vi "RT.vi"() -> ()   [LabVIEW 2012]
uses:
  Type/_RT Instrument State.ctl
  Type/RT Loop Events.ctl
  Type/_RT Parameter.ctl
  Type/_RT Active Ch.ctl
  Type/_RT Expt.ctl
  Type/_Run Mode.ctl
  Type/_RT Mass Range.ctl
  Type/_RT Res Type.ctl
  Type/_LED States.ctl
  Type/_LCD Line1 Msg.ctl
  Type/_LCD Line2 Msg.ctl
  Type/_RT LED Num.ctl
  Type/_Pump Parameter.ctl
  Type/_RW Status.ctl
  Type/_RT Serial Command.ctl
  Type/_FPGA Indicator.ctl
  _RT Global.vi
  <vilib>/FPGAPlugInAG/sbRIO-9606/niLvFpga_Open_sbRIO-9606.vi
  <vilib>/Utility/error.llb/Error Cluster From Error Code.vi
  <vilib>/rvi/errors/niLvFpgaAdjustHostInterfaceError.vi
  <vilib>/Utility/config.llb/Read Key (Boolean).vi
  <vilib>/Utility/config.llb/Read Key (String).vi
  <vilib>/Utility/config.llb/Write Key (Boolean).vi
  <vilib>/Utility/config.llb/Write Key (String).vi
  <vilib>/rvi/interface/nirviOpenFPGA/nirviOpenFPGA.xnode
  FPGA Bitfiles/FPGA9606.lvbitx
  <vilib>/rvi/interface/nirviMethod/nirviMethod.xnode
  <vilib>/rvi/interface/nirviReadWriteControl/nirviReadWriteControl.xnode
  <vilib>/Utility/config.llb/NI_LVConfig.lvlib
  <vilib>/NI_Real-Time Target Support.lvlib
  <vilib>/rvi/errors/niLvFpgaMergeErrorWithErrorCode.vi
  NiFpgaLv.dll
  <vilib>/FPGAPlugInAG/sbRIO-9606/niLvFpga_ConfigureFifo_sbRIO-9606.vi
  <vilib>/FPGAPlugInAG/sbRIO-9606/niLvFpga_StartFifo_sbRIO-9606.vi
panel:
  out "Disconnection#":u8
  out "Message Type":string
  out "Rt Loop Events":T1
  out "code":i32
  out "InstrState":T2=enum."Mass Spectrometer is Off"
  out "Fault":bool
  out "Ready":bool
  out "Running":bool
  out "RunMode":i32
  in  "RT Version":u32=965150731
  out "FPGA Version":u32
  out "Time (s)":dbl
  out "Connected?":bool
  # "Run  Status"
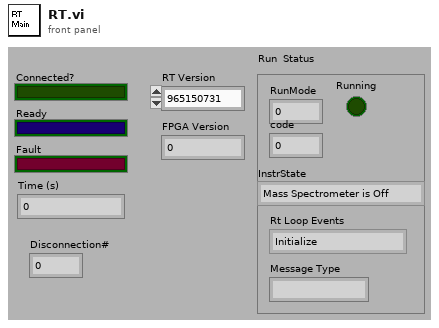
[diagram p1: front panel]
types:
  T1 = typedef "RT Loop Events.ctl" = enum16{"Initialize", "Wait for Connection", "Wait for Command", "Send Reply"}
  T2 = typedef "_RT Instrument State.ctl" = enum16{"Initializing", "Mass Spectrometer is Off", "Starting Up", "Turning Power Off", "Going to Standby", "Roughing Pump Ready", "Turning Turbo Off", "Turbo Startup", "Turbopump Ready", "Checking Vacuum", "Going to Ready", "Ready", "Running", "Source Standby", "Lost Communication", "Shutting Down", "Fault", "24V Standby", "Go to 24V Standby", "Turbopump Ready-Waiting"}
  T3 = typedef "_RT Parameter.ctl" = cluster{"RunMode":i32, "Initial Ch":T4[], "Sync":u8, "Expt":T5[], "EqTime(mS)":i32}
  T4 = typedef "_RT Active Ch.ctl" = cluster{"Start":i32, "Step":i32, "ChID":i32}
  T5 = typedef "_RT Expt.ctl" = cluster{"StartT(mS)":i32, "#Cycles":i32, "Scan Type":T6, "PauseT(uS)":i32, "Polarity":u8, "DelayT(mS)":i32, "Active Ch":T4[], "Mass Range":T7[]}
  T6 = typedef "_Run Mode.ctl" = enum16{"MRM (Q1/Q2)", "Q1 Scan", "Q1 SRM", "Q2 Scan", "Q2 SRM", "Product Scan", "Precursor Scan", "Neutral Loss", "Neutral Gain"}
  T7 = typedef "_RT Mass Range.ctl" = cluster{"Steps":i32, "Dwell(uS)":i32, "Resolution Type":T8, "Ramping Ch":T4[]}
  T8 = typedef "_RT Res Type.ctl" = u16
  T9 = typedef "Semaphore RefNum" = refnum<k1>
  T10 = typedef "_RT Instrument 2.ctl" = cluster{"Table":T11[], "Instrument":string[]}
  T11 = typedef "_RT Configuration 2.ctl" = cluster{"Name":string, "Ch#":u8, "Min":dbl, "Max":dbl, "Def+":dbl, "Def-":dbl, "Offset":dbl, "Slope":dbl, "Type":u8, "Description":string, "SettleT":dbl}
  T12 = cluster{"Rt Loop Events":T1, "Connection ID":refnum<k5>, "Parameter":T3, "Info":string, "Data Array":i32[], "error":errorcluster}
  T13 = typedef "_Pump Parameter.ctl" = enum16{"Turn Pump Motor On", "Turn Pump Motor Off", "Read Pump Oil Deficiency", "Read Rotation Switch Point Attained", "Read Ele. Drive Over Temperature", "Read Pump Over Temperature", "Read Set Rotation Speed Attained", "Read Turbopump Accelerates", "Read Actual Rotation Speed in Hz", "Read Motor Current in A", "Read Operating Hours in h", "Read Motor Voltage in V", "Read Motor Power in W", "Set Rotation Speed Switchpoint in %", "Clear Error", "Read Error Code", "Read Bearing Temperature", "Read Hardware Version", "Read Firmware Version", "Read Operating Hours (Drive)", "Read Rotational Speed (rpm)", "Read Power Stage Temperature", "Read Electronics Temperature", "Read Upper Pump Temperature", "Read Motor Temperature", "Read Error Code History, 1", "Read Error Code History, 2", "Read Error Code History, 3", "Read Error Code History, 4", "Read Error Code History, 5", "Read Error Code History, 6", "Read Error Code History, 7", "Read Error Code History, 8", "Read Error Code History, 9", "Read Error Code History, 10"}
  T14 = typedef "_RW Status.ctl" = enum8{"Done", "Do Read", "Do Write", "Set Latch1", "Set Latch2", "Set Latch3", "Set Latch4", "RP ON", "EL ON", "Serial Send", "Set LC Out", "Get LC In", "Read VAC", "Table Test", "Get Interlock", "Do Read2", "Do Write2"}
  T15 = typedef "_RT Serial Command.ctl" = cluster{"Port Type":u16, "baud rate (9600)":u32, "data bits (8)":u16, "stop bits (1)":u16, "parity (0:none)":u16, "DoRead":bool, "Command":string}
  T16 = typedef "_FPGA Indicator.ctl" = enum16{"Done", "Ready", "Count Available", "SendSerial", "LED State"}
  T17 = typedef "NI_LVConfig.lvlib/Config Data RefNum.ctl" = refnum<k1>
  T18 = typedef "_RT Startup Options.ctl" = cluster{"Door":bool, "Curtain":bool, "Pressure":bool, "Turbo":bool, "SysPoll":bool, "GasFlag":bool}
  T19 = cluster{"Info":string, "Data Array":i32[], "error":errorcluster}
  T20 = typedef "_RT LED Num.ctl" = enum8{"ReadKey", "ClearKeyBuffer", "ClearLCD", "BacklightOn"}
  T21 = typedef "_LED States.ctl" = enum8{"Idle", "Solid B", "Solid R", "Solid P", "Off B", "Off R", "Off P", "Off BRP", "Off RP", "Flash R&P", "Flash P"}
  T22 = typedef "_LCD Line2 Msg.ctl" = u16
  T23 = typedef "_LCD Line1 Msg.ctl" = u16
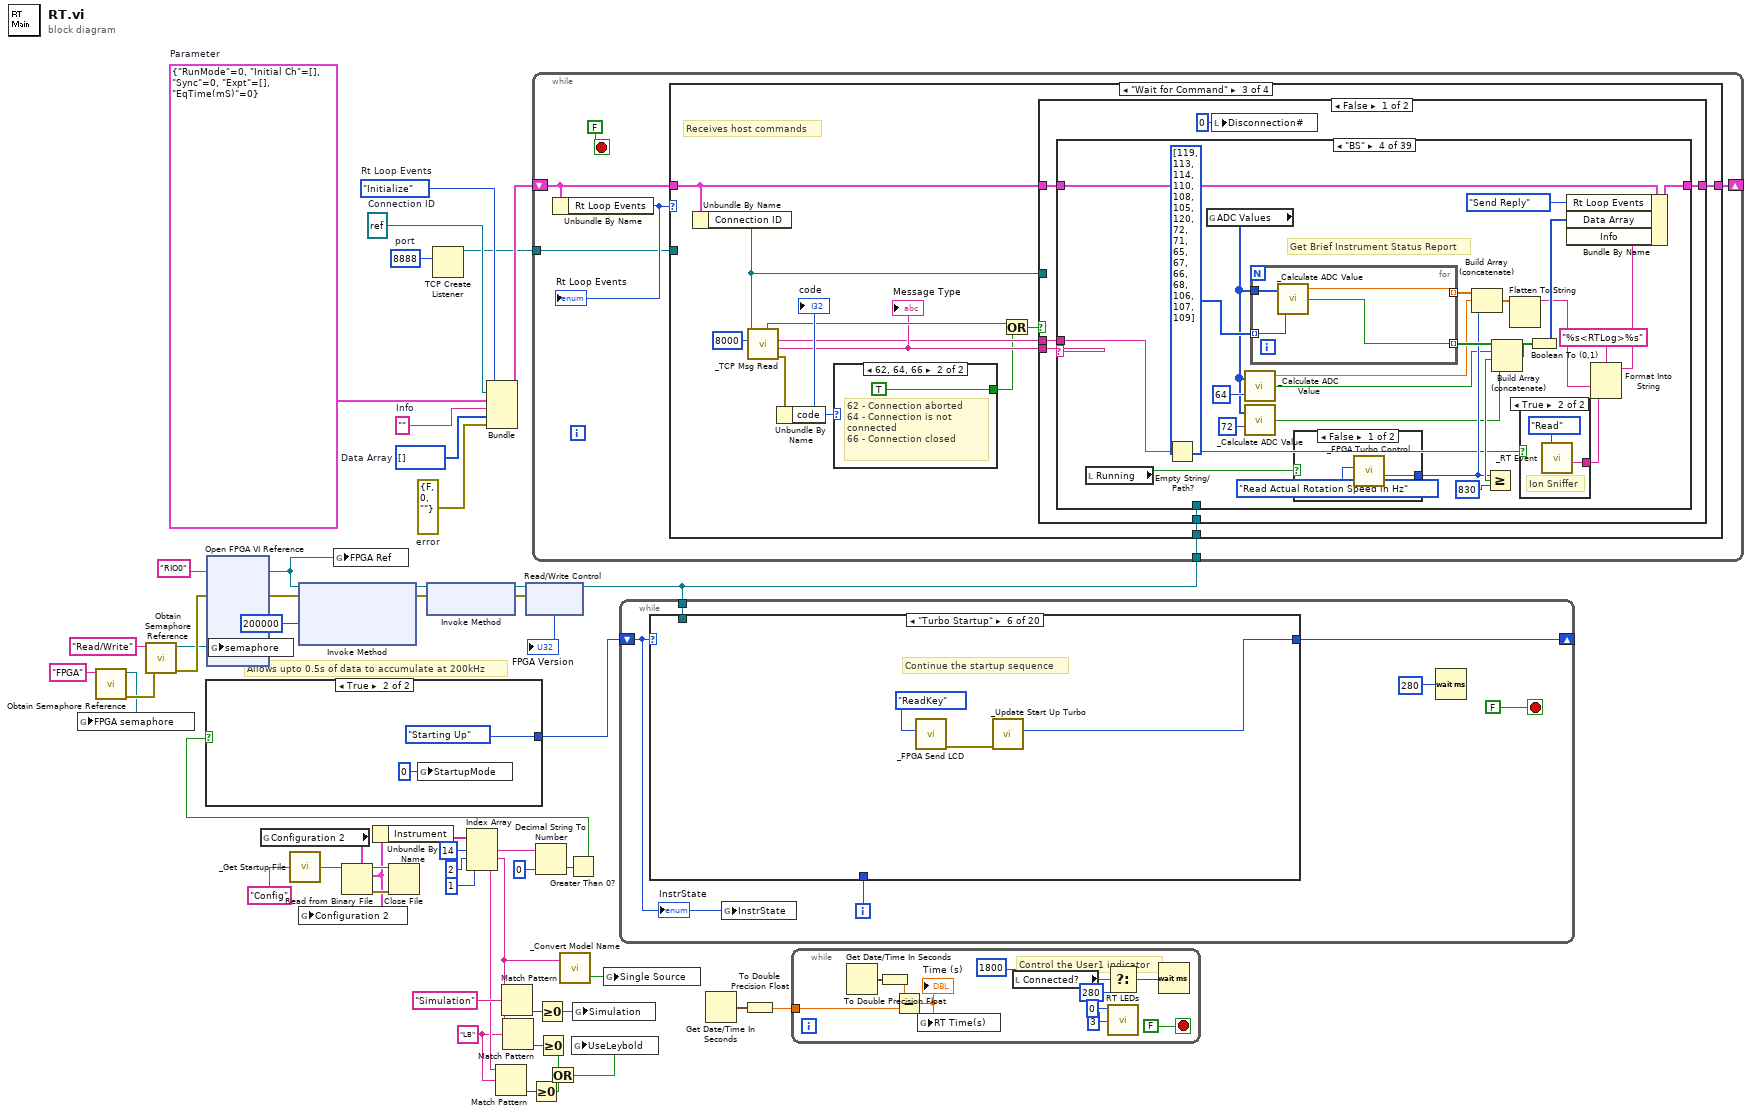
[diagram p0: block diagram]
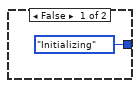
[diagram p2: hidden frame]
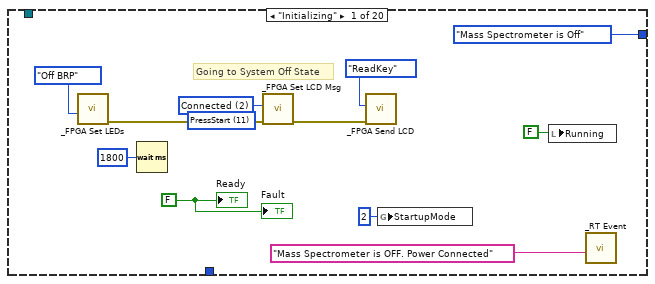
[diagram p3: hidden frame]
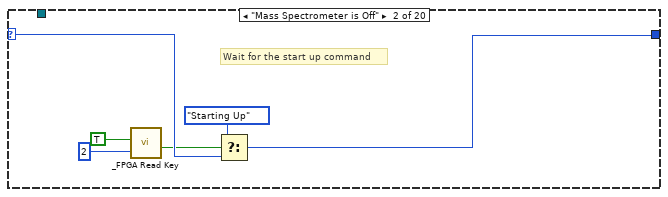
[diagram p4: hidden frame]
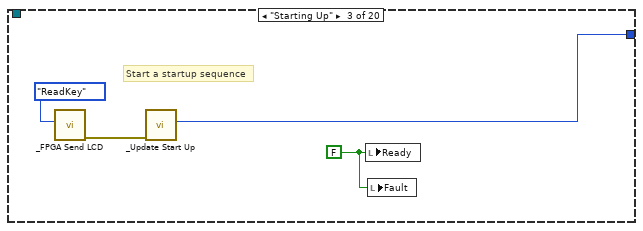
[diagram p5: hidden frame]
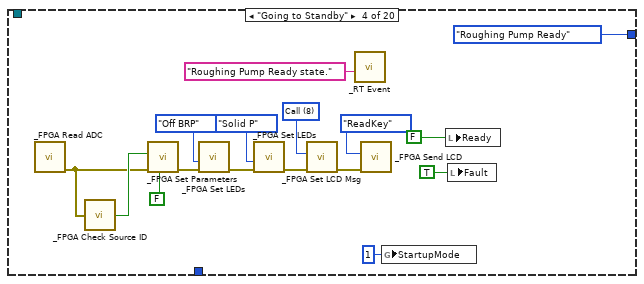
[diagram p6: hidden frame]
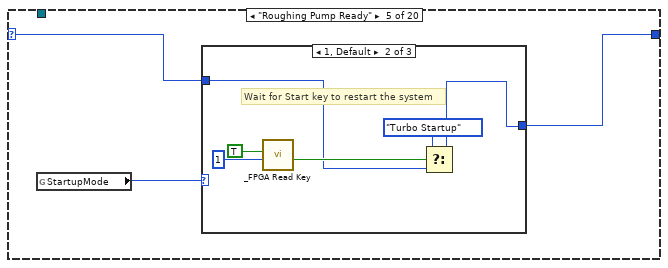
[diagram p7: hidden frame]
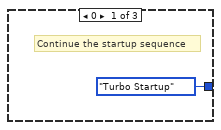
[diagram p8: hidden frame]
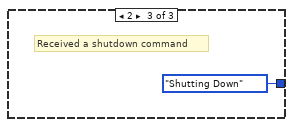
[diagram p9: hidden frame]
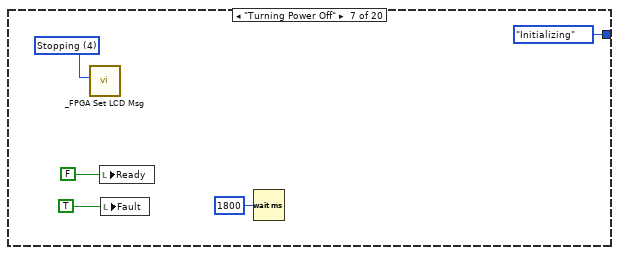
[diagram p10: hidden frame]
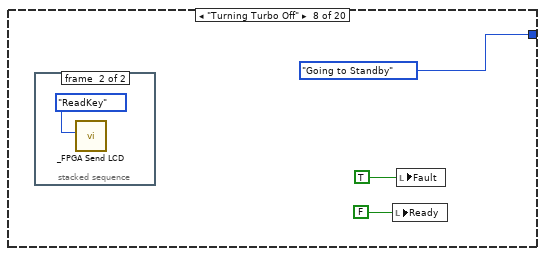
[diagram p11: hidden frame]
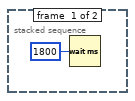
[diagram p12: hidden frame]
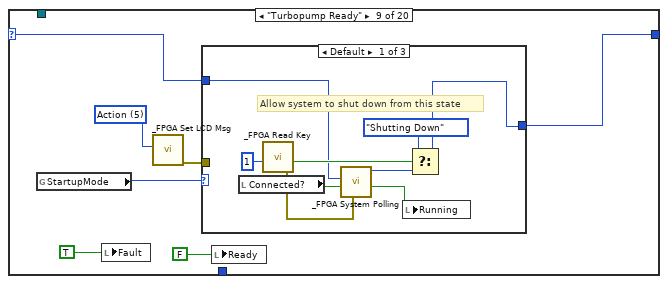
[diagram p13: hidden frame]
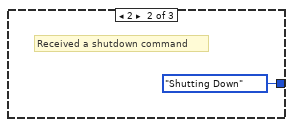
[diagram p14: hidden frame]
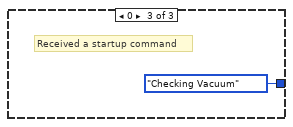
[diagram p15: hidden frame]
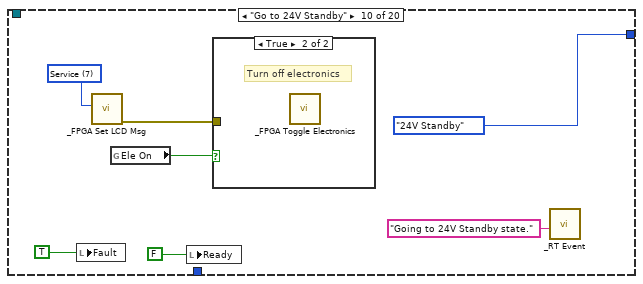
[diagram p16: hidden frame]
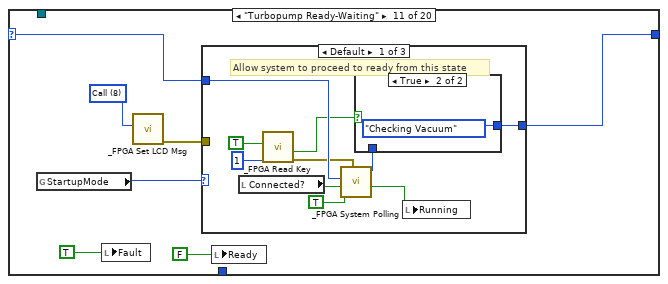
[diagram p18: hidden frame]
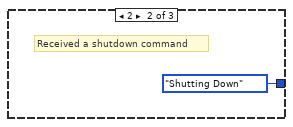
[diagram p20: hidden frame]
diagram:
  w4 = "LB" ("regular expression")
  w39 = T3 {"RunMode"=0, "Initial Ch"=[], "Sync"=0, "Expt"=[], "EqTime(mS)"=0}  # Parameter
  w41 = u16 8888  # port
  w49 = i32[] []  # Data Array
  w50 = ""  # Info
  w51 = errorcluster {"status"=FALSE, "code"=0, "source"=""}  # error
  w53 = refnum<k5> refnum  # Connection ID
  w54 = RT_Loop_Events."Initialize"  # Rt Loop Events
  # "Allows upto 0.5s of data to accumulate at 200kHz"
  n1 = call <vilib>:"Obtain Semaphore Reference.vi"("name (unnamed)"="FPGA") -> ("error out"=w23:errorcluster, "semaphore"=w21:T9)  [unwired: 2 in, 3 out]
  n2 = global write "_RT Global.vi" "FPGA semaphore"(w21) -> ()
  n3 = call <vilib>:"Obtain Semaphore Reference.vi"("error in (no error)"=w23, "name (unnamed)"="Read/Write") -> ("error out"=w26:errorcluster, "semaphore"=w25:T9)  [unwired: 1 in, 3 out]
  n4 = xnode "Open FPGA VI Reference"("error in"=w26, "resource name"="RIO0") -> ("FPGA VI Reference Out"=w12:refnum<k20>, "error out"=w43:errorcluster)
  n5 = global write "_RT Global.vi" "semaphore"(w25) -> ()
  n6 = global read "_RT Global.vi" "Configuration 2"() -> (w37:T10)
  n7 = call "_Get Startup File.vi"("FileName"="Config" ("key")) -> ("FilePath"=w11:path)
  n8 = xnode "Invoke Method"("FPGA VI Reference In"=w12, "error in"=w43, "Requested Depth"=u32 200000 ("Depth")) -> ("FPGA VI Reference Out"=w45:refnum<k20>, "error out"=w46:errorcluster)  [unwired: 1 out]
  n9 = global write "_RT Global.vi" "FPGA Ref"(w12) -> ()
  n10 = Read from Binary File(5:w37, 11:w11) -> (0:w36:errorcluster, 2:w34:T10, 3:w35:refnum<file>)  [unwired: 1 in, 4 out]
  n11 = global write "_RT Global.vi" "Configuration 2"(w34) -> ()
  n12 = Unbundle By Name(w34) -> ("Instrument"=w33:string[])
  n13 = Close File(refnum=w35, error in=w36) -> ()  [unwired: 2 out]
  n14 = xnode "Invoke Method"("FPGA VI Reference In"=w45, "error in"=w46) -> ("FPGA VI Reference Out"=w47:refnum<k20>, "error out"=w48:errorcluster)
  n15 = TCP Create Listener(10:w41) -> (3:w40:refnum<k5>)  [unwired: 1 in, 5 out]
  n16 = Index Array(array=w33, index #1=14 ("index"), index #2=2 ("index"), index #3=1 ("index")) -> (element #1=w30:string, element #2=w8:string, element #3=w5:string)
  n17 = Bundle("Rt Loop Events"=w54, "Connection ID"=w53, "Parameter"=w39, "Info"=w50, "Data Array"=w49, "error"=w51) -> (w52:T12)  [unwired: 1 out]
  n18 = Match Pattern(string=w5, regular expression=w4) -> (offset past match=w6:i32)  [unwired: 4 out]
  n19 = Match Pattern(string=w8, regular expression="Simulation") -> (offset past match=w19:i32)  [unwired: 4 out]
  n20 = Match Pattern(string=w8, regular expression=w4) -> (offset past match=w9:i32)  [unwired: 4 out]
  n21 = xnode "Read/Write Control"("FPGA VI Reference In"=w47, "error in"=w48) -> ("FPGA VI Reference Out"=w15:refnum<k20>, "Version"=→"FPGA Version":u32)  [unwired: 1 out]
  n22 = Greater Or Equal To 0?(x=w6) -> (x >= 0?=w2:bool)
  n23 = while {
    shift-right: [w57] -> _
    shift-left: w52 -> [w58]
    tunnel: w15 -> [w56]
    tunnel: w40 -> [w55]
    stop <- FALSE stop-if-true
    n24 = Unbundle By Name(w58) -> ("Rt Loop Events"=w59:T1)
    "Rt Loop Events" <- w59
    n25 = case shown="\"Wait for Command\"" w59 {
      tunnel: w58 -> [w85 w126 w146 w778]
      tunnel: [w84 w125 w145 w777] -> w57
      tunnel: w56 -> [_ _ w141 _]
      tunnel: w55 -> [_ w123 _ _]
      frame "Initialize", Default {
        w63 = FALSE ("Connected?")
        w78 = FALSE ("Connected?")
        w73 = "RT" ("section")
        # "Initialize All Instrument Parameters"
        n26 = stacked-sequence {
          frame #0 {
            n27 = call "_Read RT Table.vi"("key"="Cal") -> ("Table"=w87:dbl[][])  [unwired: 2 in, 4 out]
            n28 = global write "_RT Global.vi" "Q1 Cal"(w87) -> ()
            n29 = call "_Read RT Table.vi"("key"="Cal2") -> ("Table"=w88:dbl[][])  [unwired: 2 in, 4 out]
            n30 = global write "_RT Global.vi" "Q2 Cal"(w88) -> ()
            n31 = call "_Read RT Table.vi"("key"="Cal3") -> ("Table"=w89:dbl[][])  [unwired: 2 in, 4 out]
            n32 = global write "_RT Global.vi" "Q1 -Cal"(w89) -> ()
            n33 = call "_Read RT Table.vi"("key"="Cal4") -> ("Table"=w90:dbl[][])  [unwired: 2 in, 4 out]
            n34 = global write "_RT Global.vi" "Q2 -Cal"(w90) -> ()
            n35 = call "_Read RT Table.vi"("key"="Res") -> ("Table"=w91:dbl[][])  [unwired: 2 in, 4 out]
            n36 = global write "_RT Global.vi" "Q1 Res Hi"(w91) -> ()
            n37 = call "_Read RT Table.vi"("key"="Res2") -> ("Table"=w92:dbl[][])  [unwired: 2 in, 4 out]
            n38 = global write "_RT Global.vi" "Q2 Res Hi"(w92) -> ()
            n39 = call "_Read RT Table.vi"("key"="Res3") -> ("Table"=w93:dbl[][])  [unwired: 2 in, 4 out]
            n40 = global write "_RT Global.vi" "Q1 Res Med"(w93) -> ()
            n41 = call "_Read RT Table.vi"("key"="Res4") -> ("Table"=w94:dbl[][])  [unwired: 2 in, 4 out]
            n42 = global write "_RT Global.vi" "Q2 Res Med"(w94) -> ()
            n43 = call "_Read RT Table.vi"("key"="Res5") -> ("Table"=w95:dbl[][])  [unwired: 2 in, 4 out]
            n44 = global write "_RT Global.vi" "Q1 Res Lo"(w95) -> ()
            n45 = call "_Read RT Table.vi"("key"="Res6") -> ("Table"=w96:dbl[][])  [unwired: 2 in, 4 out]
            n46 = global write "_RT Global.vi" "Q2 Res Lo"(w96) -> ()
            n47 = call "_Read RT Table.vi"("key"="Res7") -> ("Table"=w97:dbl[][])  [unwired: 2 in, 4 out]
            n48 = global write "_RT Global.vi" "Q1 -Res Hi"(w97) -> ()
            n49 = call "_Read RT Table.vi"("key"="Res8") -> ("Table"=w98:dbl[][])  [unwired: 2 in, 4 out]
            n50 = global write "_RT Global.vi" "Q2 -Res Hi"(w98) -> ()
            n51 = call "_Read RT Table.vi"("key"="Res9") -> ("Table"=w99:dbl[][])  [unwired: 2 in, 4 out]
            n52 = global write "_RT Global.vi" "Q1 -Res Med"(w99) -> ()
            n53 = call "_Read RT Table.vi"("key"="Res10") -> ("Table"=w100:dbl[][])  [unwired: 2 in, 4 out]
            n54 = global write "_RT Global.vi" "Q2 -Res Med"(w100) -> ()
            n55 = call "_Read RT Table.vi"("key"="Res11") -> ("Table"=w101:dbl[][])  [unwired: 2 in, 4 out]
            n56 = global write "_RT Global.vi" "Q1 -Res Lo"(w101) -> ()
            n57 = call "_Read RT Table.vi"("key"="Res12") -> ("Table"=w102:dbl[][])  [unwired: 2 in, 4 out]
            n58 = global write "_RT Global.vi" "Q2 -Res Lo"(w102) -> ()
          }
          frame #1 {
            n59 = for {
              N: 16 -> [_]
              i -> [w120]
              n60 = call "_Update Cal or Res Data.vi"("Table Type"=w120) -> ()  [unwired: 2 in, 5 out]
            }
          }
        }
        n61 = call "_Get Startup File.vi"("FileName"="ADC" ("key")) -> ("FilePath"=w62:path)
        n62 = global read "_RT Global.vi" "ADC Table"() -> (w64:T11[])
        n63 = Read from Binary File(5:w64, 11:w62) -> (0:w66:errorcluster, 2:w65:T11[], 3:w67:refnum<file>)  [unwired: 1 in, 4 out]
        n64 = global write "_RT Global.vi" "ADC Table"(w65) -> ()
        n65 = Close File(refnum=w67, error in=w66) -> ()  [unwired: 2 out]
        n66 = Bundle By Name(cluster=w85, "Rt Loop Events"=RT_Loop_Events."Wait for Connection") -> (w84:T12)
        n67 = call "_RT Open Preference File.vi"() -> ("refnum"=w77:T17)  [unwired: 7 out]
        n68 = global read "_RT Global.vi" "StartupOptions"() -> (w68:T18)
        n69 = local write "Connected?"(w63) -> ()
        n70 = local write "Ready"(w63) -> ()
        n71 = call-poly <vilib>:"Read Key.vi"("section"=w73, "default value"=w78, "key"="Q1Pol", "refnum"=w77) -> ("value"=w79:bool, "refnum out"=w80:T17)  [unwired: 1 in, 5 out]
        n72 = local write "Fault"(w63) -> ()
        n73 = global write "_RT Global.vi" "IgnoreError"(w63) -> ()
        n74 = global write "_RT Global.vi" "Ele On"(w63) -> ()
        n75 = Flatten To String(anything=w68) -> (data string=w71:string)  [unwired: 1 in, 4 out]
        n76 = call-poly <vilib>:"Read Key.vi"("section"=w73, "default value"=w78, "key"="Q2Pol", "refnum"=w80) -> ("value"=w76:bool, "refnum out"=w75:T17)  [unwired: 1 in, 5 out]
        n77 = global write "_RT Global.vi" "Q2 POL"(w76) -> ()
        n78 = global write "_RT Global.vi" "Q1 POL"(w79) -> ()
        n79 = call-poly <vilib>:"Read Key.vi"("section"=w73, "default value"=w71, "key"="SUOpt", "refnum"=w75) -> ("value"=w70:string, "refnum out"=w72:T17)  [unwired: 2 in, 4 out]
        n80 = Unflatten From String(type=w68, binary string=w70) -> (value=w69:T18)  [unwired: 1 in, 4 out]
        n81 = global write "_RT Global.vi" "StartupOptions"(w69) -> ()
        n82 = call <vilib>:"Close Config Data.vi"("write file if changed (T)"=TRUE ("write configuration file? (T)"), "refnum"=w72) -> ()  [unwired: 1 in, 9 out]
      }
      frame "Wait for Connection" {
        # "Waits for new host connection"
        n83 = TCP Wait On Listener(9:-1 ("timeout ms (wait forever: -1)"), 11:w123) -> (0:w124:errorcluster, 4:w122:refnum<k5>)  [unwired: 1 in, 4 out]
        n84 = case shown="No Error" w124 {
          tunnel: w126 -> [w133 w136]
          tunnel: w122 -> [w130 _]
          tunnel: [w132 w134] -> w125
          frame No Error {
            n85 = local write "Disconnection#"(u8 0 ("Disconnection#")) -> ()
            n86 = local write "Connected?"(TRUE ("Connected?")) -> ()
            n87 = call "_RT Event.vi"("Event"="PC Communication Established") -> ()  [unwired: 2 in, 5 out]
            n88 = Bundle By Name(cluster=w133, "Connection ID"=w130, "Rt Loop Events"=RT_Loop_Events."Wait for Command") -> (w132:T12)
          }
          frame Error {
            n89 = Bundle By Name(cluster=w136, "Rt Loop Events"=RT_Loop_Events."Wait for Connection") -> (w134:T12)
          }
        }
      }
      frame "Wait for Command" {
        # "Receives host commands"
        n90 = Unbundle By Name(w146) -> ("Connection ID"=w138:refnum<k5>)
        n91 = call "_TCP Msg Read.vi"("timeout ms (10000)"=8000 ("millisecond multiple"), "connection ID"=w138) -> ("error out"=w140:errorcluster, "Message Type"=w144:string, "Data Stream"=w143:string, "Timed Out?"=w147:bool)  [unwired: 3 in, 3 out]
        "Message Type" <- w144
        n92 = Unbundle By Name(w140) -> ("code"=w148:i32)
        "code" <- w148
        n93 = case shown="62, 64, 66" w148 {
          tunnel: [_ TRUE ("abort (F)")] -> w137
          frame Default {
          }
          frame 62, 64, 66 {
            # "62 - Connection aborted\n64 - Connection is not connected\n66 - Connection closed"
          }
        }
        n94 = Or(x=w147, y=w137) -> (x .or. y?=w139:bool)
        n95 = case shown="False" w139 {
          tunnel: w146 -> [w153 w763]
          tunnel: [w152 w762] -> w145
          tunnel: w144 -> [w150 _]
          tunnel: w143 -> [w154 _]
          tunnel: w141 -> [w151 _]
          tunnel: w138 -> [_ w759]
          frame False {
            n96 = case shown="\"BS\"" w150 {
              selector: w150 -> [_ _ _ _ _ _ _ _ _ _ _ _ _ _ _ _ _ _ _ _ _ _ _ _ _ _ _ _ _ _ _ _ _ _ _ _ _ _ w755]
              tunnel: w154 -> [_ w171 w176 w189 w221 w230 w252 w272 _ w292 _ _ _ _ _ w360 _ w425 w449 w458 _ w464 w482 w490 w498 _ w507 w531 w546 _ w575 w578 w588 w608 w628 w644 w691 w705 _]
              tunnel: w153 -> [w159 w168 w181 w206 w224 w233 w249 w269 w286 w294 w300 w305 w314 w349 w357 w364 w422 w429 w452 w455 w462 w474 w479 w487 w495 w505 w512 w534 w544 w556 w572 w582 w595 w606 w626 w641 w701 w711 w751]
              tunnel: [w158 w167 w180 w205 w223 w232 w248 w268 w285 w293 w299 w304 w313 w348 w356 w363 w421 w428 w451 w454 w461 w473 w478 w486 w494 w504 w511 w533 w543 w555 w571 w581 w594 w605 w625 w640 w700 w708 w750] -> w152
              tunnel: w151 -> [_ _ _ _ _ _ _ _ _ _ _ _ w306 w345 _ _ w418 _ _ _ _ _ _ _ _ _ _ _ w542 _ _ _ w593 w604 w624 w637 w690 _ _]
              frame "AG" {
                # "Get ADC Table"
                n97 = global read "_RT Global.vi" "ADC Table"() -> (w156:T11[])
                n98 = Flatten To String(anything=w156) -> (data string=w155:string)  [unwired: 1 in, 4 out]
                n99 = Bundle By Name(cluster=w159, "Rt Loop Events"=RT_Loop_Events."Send Reply", "Info"=w155) -> (w158:T12)
              }
              frame "AS" {
                # "Set ADC Table"
                n100 = global read "_RT Global.vi" "ADC Table"() -> (w170:T11[])
                n101 = Unflatten From String(type=w170, binary string=w171) -> (value=w166:T11[], error out=w163:errorcluster)  [unwired: 1 in, 3 out]
                n102 = call "_Get Startup File.vi"("FileName"="ADC" ("key")) -> ("FilePath"=w161:path)
                n103 = global write "_RT Global.vi" "ADC Table"(w166) -> ()
                n104 = Write to Binary File(file (use dialog)=w161, data=w166, error in=w163) -> (refnum out=w164:refnum<file>, error out=w165:errorcluster)  [unwired: 4 out]
                n105 = Close File(refnum=w164, error in=w165) -> (error out=w162:errorcluster)  [unwired: 1 out]
                n106 = Unbundle By Name(w162) -> ()  [unwired: 1 out]
                n107 = Bundle By Name(cluster=w168, "Rt Loop Events"=RT_Loop_Events."Send Reply", "error"=w162) -> (w167:T12)
              }
              frame "AU" {
                # "Send auxiliary update command"
                n108 = Scan From String(format string="%d,%f", input string=w176, default 1=-1 ("default value 1"), default 2=sgl 0.0 ("default value 2")) -> (output 1=w175:i32, output 2=w174:sgl)  [unwired: 2 in, 3 out]
                n109 = call "_FPGA Auxiliary Update.vi"("Setting Value"=w174, "Command Type"=w175) -> ("error out"=w173:errorcluster, "Return Value"=w172:string)  [unwired: 1 in, 3 out]
                n110 = Bundle By Name(cluster=w181, "Rt Loop Events"=RT_Loop_Events."Send Reply", "Info"=w172, "error"=w173) -> (w180:T12)
              }
              frame "BS" {
                # "Get Brief Instrument Status Report"
                n111 = local read "Running"() -> (w183:bool)
                n112 = Empty String/Path?(string/path=w189) -> (empty?=w188:bool)
                n113 = global read "_RT Global.vi" "ADC Values"() -> (w186:i32[])
                n114 = call "_Calculate ADC Value.vi"("ADC Values"=w186, "ADC Channel (64)"=u8 64) -> ("User Value"=w194:sgl, "In Range?"=w185:bool)  [unwired: 1 out]
                n115 = call "_Calculate ADC Value.vi"("ADC Values"=w186, "ADC Channel (64)"=u8 72) -> ("In Range?"=w184:bool)  [unwired: 2 out]
                n116 = for {
                  tunnel: i32[] [119, 113, 114, 110, 108, 105, 120, 72, 71, 65, 67, 66, 68, 106, 107, 109] -> [w215] mode=indexing
                  tunnel: w186 -> [w216]
                  tunnel: [w214] -> w201 mode=indexing
                  tunnel: [w213] -> w203 mode=indexing
                  n117 = call "_Calculate ADC Value.vi"("ADC Values"=w216, "ADC Channel (64)"=w215) -> ("User Value"=w214:sgl, "In Range?"=w213:bool)  [unwired: 1 out]
                }
                n118 = case shown="False" w183 {
                  tunnel: [w208 830 ("Speed")] -> w196
                  frame False {
                    n119 = call "_FPGA Turbo Control.vi"("Command"=_Pump_Parameter."Read Actual Rotation Speed in Hz") -> ("Speed"=w208:i32)  [unwired: 3 in, 5 out]
                  }
                  frame True {
                  }
                }
                n120 = Build Array (concatenate)(w201, w194, w196) -> (w197:sgl[])
                n121 = Greater Or Equal?(x=w196, y=830) -> (x >= y?=w198:bool)
                n122 = Build Array (concatenate)(w203, w185, w198, w184) -> (w199:bool[])
                n123 = Flatten To String(anything=w197) -> (data string=w191:string)  [unwired: 1 in, 4 out]
                n124 = case shown="True" w188 {
                  tunnel: [_ w211] -> w193
                  frame False {
                    # "for Server"
                  }
                  frame True {
                    # "Ion Sniffer"
                    n125 = call "_RT Event.vi"("Action (Write)"=enum16{"Write", "Read"}."Read") -> ("Log"=w211:string)  [unwired: 2 in, 4 out]
                  }
                }
                n126 = Boolean To (0,1)(Boolean=w199) -> (0, 1=w202:i16[])
                n127 = Format Into String(format string="%s<RTLog>%s", w191, w193) -> (resulting string=w190:string)  [unwired: 2 in, 1 out]
                n128 = Bundle By Name(cluster=w206, "Rt Loop Events"=RT_Loop_Events."Send Reply", "Data Array"=w202, "Info"=w190) -> (w205:T12)
              }
              frame "CC" {
                # "Set contact closure output logics:\n0 for Shimadzu; 1 for others"
                n129 = Type Cast(type=u16 0, x=w221) -> (*(type *) &x=w218:u16)
                n130 = call "_FPGA Write Data.vi"("Write Mode (Do Write)"=_RW_Status."Do Write", "Data"=w218, "Address"=u16 399) -> ("error out"=w217:errorcluster)  [unwired: 3 in, 2 out]
                n131 = Bundle By Name(cluster=w224, "Rt Loop Events"=RT_Loop_Events."Send Reply", "error"=w217) -> (w223:T12)
              }
              frame "CI" {
                # "Set contact closure input logics:\nOption    LC1        LC2\n     0        High      High\n     1        Low        High\n     2        High       Low\n     3        Low        Low"
                n132 = Type Cast(type=u16 0, x=w230) -> (*(type *) &x=w227:u16)
                n133 = call "_FPGA Write Data.vi"("Write Mode (Do Write)"=_RW_Status."Do Write", "Data"=w227, "Address"=u16 409) -> ("error out"=w226:errorcluster)  [unwired: 3 in, 2 out]
                n134 = Bundle By Name(cluster=w233, "Rt Loop Events"=RT_Loop_Events."Send Reply", "error"=w226) -> (w232:T12)
              }
              frame "CP" {
                # "Set Source Polarity:"
                # "Set CEM POL for Latch4"
                # "Set S1 POL, S2 POL for Latch3"
                # "Set COR POL, CUR POL for Latch2"
                n135 = Type Cast(type=u16 0, x=w252) -> (*(type *) &x=w237:u16)
                n136 = Greater Than 0?(x=w237) -> (x > 0?=w236:bool)
                n137 = Number To Boolean Array(number=u16 0) -> (Boolean array=w241:bool[])
                n138 = Replace Array Subset(array=w241, new element #1=w236, index #1=0 ("index"), new element #2=w236, index #2=1 ("index")) -> (w238:bool[])
                n139 = Boolean Array To Number(Boolean array=w238) -> (number=w235:u16)
                n140 = call "_FPGA Set Digi Line.vi"("States"=w235, "Line (Set Latch1)"=_RW_Status."Set Latch2" ("Write Mode (Do Write)")) -> ("error out"=w246:errorcluster)  [unwired: 2 in, 3 out]
                n141 = call "_FPGA Set Digi Line.vi"("error in"=w246, "States"=w235, "Line (Set Latch1)"=_RW_Status."Set Latch3" ("Write Mode (Do Write)")) -> ("error out"=w244:errorcluster)  [unwired: 1 in, 3 out]
                n142 = call "_FPGA Set Digi Line.vi"("error in"=w244, "States"=w235, "Line (Set Latch1)"=_RW_Status."Set Latch4" ("Write Mode (Do Write)")) -> ("error out"=w243:errorcluster)  [unwired: 1 in, 3 out]
                n143 = Bundle By Name(cluster=w249, "Rt Loop Events"=RT_Loop_Events."Send Reply", "error"=w243) -> (w248:T12)
              }
              frame "DP" {
                w257 = "RT" ("section")
                # "Set Q1 POL, Q2 POL, Q1DC EN, Q2DC EN"
                n144 = Type Cast(type=u16 0, x=w272) -> (*(type *) &x=w266:u16)
                n145 = Number To Boolean Array(number=w266) -> (Boolean array=w265:bool[])
                n146 = call "_FPGA Set Digi Line.vi"("States"=w266, "Line (Set Latch1)"=_RW_Status."Set Latch1" ("Write Mode (Do Write)")) -> ("error out"=w267:errorcluster)  [unwired: 2 in, 3 out]
                n147 = Index Array(array=w265) -> (element #1=w255:bool, element #2=w254:bool)  [unwired: 2 in]
                n148 = global write "_RT Global.vi" "Q1 POL"(w255) -> ()
                n149 = global write "_RT Global.vi" "Q2 POL"(w254) -> ()
                n150 = call "_RT Open Preference File.vi"() -> ("error"=w262:errorcluster, "refnum"=w261:T17)  [unwired: 6 out]
                n151 = call-poly <vilib>:"Write Key.vi"("section"=w257, "error in (no error)"=w262, "value"=w255, "key"="Q1Pol", "refnum"=w261) -> ("error out"=w259:errorcluster, "refnum out"=w258:T17)  [unwired: 5 out]
                n152 = call-poly <vilib>:"Write Key.vi"("section"=w257, "error in (no error)"=w259, "value"=w254, "key"="Q2Pol", "refnum"=w258) -> ("error out"=w264:errorcluster, "refnum out"=w263:T17)  [unwired: 5 out]
                n153 = call <vilib>:"Close Config Data.vi"("error in (no error)"=w264, "refnum"=w263) -> ()  [unwired: 1 in, 9 out]
                n154 = Bundle By Name(cluster=w269, "Rt Loop Events"=RT_Loop_Events."Send Reply", "error"=w267) -> (w268:T12)
              }
              frame "DS" {
                # "Get Detailed Instrument Status Report"
                n155 = local read "Running"() -> (w280:bool)
                n156 = local read "Ready"() -> (w281:bool)
                n157 = local read "Fault"() -> (w277:bool)
                n158 = Select(t="1", s=w280, f="0") -> (s? t:f=w282:string)
                n159 = Select(t=w282, s=w281, f="2") -> (s? t:f=w283:string)
                n160 = Select(t="3", s=w277, f=w283) -> (s? t:f=w276:string)
                n161 = call "_FPGA Get System Status.vi"("Server State"=w276) -> ("Status"=w284:string)  [unwired: 1 in, 5 out]
                n162 = Bundle By Name(cluster=w286, "Rt Loop Events"=RT_Loop_Events."Send Reply", "Info"=w284) -> (w285:T12)
              }
              frame "EL" {
                # "Toggle Electrics"
                n163 = Not Equal?(x=w292, y="0") -> (x != y?=w290:bool)
                n164 = Boolean To (0,1)(Boolean=w290) -> (0, 1=w289:i16)
                n165 = call "_FPGA Toggle Electronics.vi"("Ele On (1 for ON and 0 for OFF)"=w289) -> ("error out"=w288:errorcluster)  [unwired: 2 in, 5 out]
                n166 = Bundle By Name(cluster=w294, "Rt Loop Events"=RT_Loop_Events."Send Reply", "error"=w288) -> (w293:T12)
              }
              frame "EN" {
                w297 = u16 0 ("Address")
                # "End a Run"
                n167 = call "_FPGA Write Data.vi"("Data"=w297, "Address"=w297) -> ("error out"=w296:errorcluster)  [unwired: 4 in, 2 out]
                n168 = Bundle By Name(cluster=w300, "Rt Loop Events"=RT_Loop_Events."Send Reply", "error"=w296) -> (w299:T12)
              }
              frame "GC" {
                # "Get Configuration"
                n169 = global read "_RT Global.vi" "Configuration 2"() -> (w302:T10)
                n170 = Flatten To String(anything=w302) -> (data string=w301:string)  [unwired: 1 in, 4 out]
                n171 = Bundle By Name(cluster=w305, "Rt Loop Events"=RT_Loop_Events."Send Reply", "Info"=w301) -> (w304:T12)
              }
              frame "GD" {
                # "Get data and check for FPGA status"
                n172 = xnode "Read/Write Control"("FPGA VI Reference In"=w306) -> ("error out"=w308:errorcluster, "Running"=w311:bool)  [unwired: 1 in, 1 out]
                n173 = local write "Running"(w311) -> ()
                n174 = case shown="No Error" w308 {
                  selector: w308 -> [w316 w322]
                  tunnel: [w318 _] -> w309
                  tunnel: [w317 _] -> w310
                  tunnel: [w315 w320] -> w307
                  frame No Error {
                    n175 = call "_FPGA Read Counter.vi"("error in (no error)"=w316) -> ("error out"=w315:errorcluster, "size(s)"=w319:u32, "Data"=w317:i32[])  [unwired: 1 in, 1 out]
                    n176 = Number To Decimal String(number=w319) -> (decimal integer string=w318:string)  [unwired: 1 out]
                  }
                  frame Error {
                    n177 = call "_Construct Error Cluster.vi"("error in"=w322, "reason"="Engine Error:\nFound while getting data and checking FPGA status.") -> ("error out"=w320:errorcluster)  [unwired: 2 in, 3 out]
                  }
                }
                n178 = Bundle By Name(cluster=w314, "Rt Loop Events"=RT_Loop_Events."Send Reply", "Info"=w309, "Data Array"=w310, "error"=w307) -> (w313:T12)
              }
              frame "GI" {
                w336 = u32 60 ("y")
                # "Get Info"
                n179 = local read "Time (s)"() -> (w332:dbl)
                n180 = xnode "Read/Write Control"("FPGA VI Reference In"=w345) -> ("FPGA VI Reference Out"=w342:refnum<k20>, "error out"=w343:errorcluster, "Version"=w344:u32)  [unwired: 1 in]
                n181 = local read "Ready"() -> (w329:bool)
                n182 = xnode "Read/Write Control"("FPGA VI Reference In"=w342, "error in"=w343) -> ("Running"=w330:bool)  [unwired: 2 out]
                n183 = local write "Running"(w330) -> ()
                n184 = Select(t="System is running", s=w330, f="System is idling") -> (s? t:f=w327:string)
                n185 = To Unsigned Long Integer(number=w332) -> (unsigned 32bit integer=w334:u32)
                n186 = local read "Fault"() -> (w325:bool)
                n187 = Quotient & Remainder(x=w334, y=w336) -> (x-y*floor(x/y)=w337:u32, floor(x/y)=w335:u32)
                n188 = Select(t=w327, s=w329, f="System is not ready.") -> (s? t:f=w324:string)
                n189 = Select(t="System is in a fault state.", s=w325, f=w324) -> (s? t:f=w323:string)
                n190 = Quotient & Remainder(x=w335, y=w336) -> (x-y*floor(x/y)=w338:u32, floor(x/y)=w339:u32)
                n191 = Format Into String(format string="Ionica Firmware; FPGA: %d; RT: %d\n(%s: %dh%dm%ds)", w344, "RT Version", w323, w339, w338, w337) -> (resulting string=w346:string)  [unwired: 2 in, 1 out]
                n192 = Bundle By Name(cluster=w349, "Rt Loop Events"=RT_Loop_Events."Send Reply", "Info"=w346) -> (w348:T12)
              }
              frame "GL" {
                # "Get LC Inputs"
                n193 = call "_FPGA Read Data.vi"("Read Mode (Do Read)"=_RW_Status."Get LC In" ("R/W Status")) -> ("error out"=w350:errorcluster, "Data"=w351:u32)  [unwired: 4 in, 1 out]
                n194 = Split Number(x=w351) -> (hi(x)=w355:u16, lo(x)=w354:u16)
                n195 = Build Array(w355, w354) -> (w353:u16[])
                n196 = Bundle By Name(cluster=w357, "Rt Loop Events"=RT_Loop_Events."Send Reply", "Data Array"=w353, "error"=w350) -> (w356:T12)
              }
              frame "GP" {
                n197 = Decimal String To Number(string=w360) -> (number=w359:i32)  [unwired: 3 out]
                n198 = case shown="0" w359 {
                  selector: w359 -> [_ w371]
                  tunnel: [w365 w367] -> w361
                  frame 0 {
                    # "Get Parameter"
                    n199 = call "_Get FPGA Info.vi"() -> ("Info"=w365:string)  [unwired: 2 in, 5 out]
                  }
                  frame 1, Default {
                    # "Get Cal/Res Table"
                    n200 = Decrement(x=w371) -> (x-1=w370:i32)
                    n201 = case shown="13" w370 {
                      tunnel: [u16 500 ("Addr Offset") u16 550 ("Addr Offset") u16 600 ("Addr Offset") u16 650 ("Addr Offset") u16 700 ("Addr Offset") u16 750 ("Addr Offset") u16 800 ("Addr Offset") u16 850 ("Addr Offset") u16 900 ("Addr Offset") u16 950 ("Addr Offset") u16 1000 ("Addr Offset") u16 1050 ("Addr Offset") u16 1100 ("Addr Offset") u16 1150 ("Addr Offset") u16 1200 ("Addr Offset") u16 1250 ("Addr Offset")] -> w368
                      frame 0, Default {
                      }
                      frame 1 {
                      }
                      frame 2 {
                      }
                      frame 3 {
                      }
                      frame 4 {
                      }
                      frame 5 {
                      }
                      frame 6 {
                      }
                      frame 7 {
                      }
                      frame 8 {
                      }
                      frame 9 {
                      }
                      frame 10 {
                      }
                      frame 11 {
                      }
                      frame 12 {
                      }
                      frame 13 {
                      }
                      frame 14 {
                      }
                      frame 15 {
                      }
                    }
                    n202 = for {
                      N: 25 -> [_]
                      shift-right: [w377] -> w367
                      shift-left: "" -> [w380]
                      tunnel: w368 -> [w384]
                      shift-right: [w381] -> _
                      shift-left: _ -> [w382]
                      i -> [w387]
                      # "For each row"
                      n203 = Multiply(x=w387, y=2) -> (x*y=w385:i32)
                      n204 = Add(x=w385, y=w384) -> (x+y=w379:i32)
                      n205 = call "_FPGA Read Data.vi"("error in"=w382, "Address"=w379) -> ("error out"=w383:errorcluster, "Data"=w378:u32)  [unwired: 3 in, 1 out]
                      n206 = Increment(x=w379) -> (x+1=w375:i32)
                      n207 = call "_Format Memory Map String.vi"("User value"="Mass Value", "Data"=w378, "Address"=w379, "String In"=w380) -> ("String Out"=w376:string)  [unwired: 3 out]
                      n208 = call "_FPGA Read Data.vi"("error in"=w383, "Address"=w375) -> ("error out"=w381:errorcluster, "Data"=w374:u32)  [unwired: 3 in, 1 out]
                      n209 = call "_Format Memory Map String.vi"("User value"="DAC Value", "Data"=w374, "Address"=w375, "String In"=w376) -> ("String Out"=w377:string)  [unwired: 3 out]
                    }
                  }
                }
                n210 = Bundle By Name(cluster=w364, "Rt Loop Events"=RT_Loop_Events."Send Reply", "Info"=w361) -> (w363:T12)
              }
              frame "GS" {
                # "Get Status"
                n211 = xnode "Read/Write Control"("FPGA VI Reference In"=w418) -> ("Running"=w417:bool)  [unwired: 1 in, 2 out]
                n212 = local read "Ready"() -> (w416:bool)
                n213 = local write "Running"(w417) -> ()
                n214 = global read "_RT Global.vi" "InstrState"() -> (w406:T2)
                n215 = Select(t="1: The system is running", s=w417, f="0: The system is idling") -> (s? t:f=w413:string)
                n216 = local read "Fault"() -> (w414:bool)
                n217 = Select(t=w413, s=w416, f="2: The system is not ready") -> (s? t:f=w412:string)
                n218 = To Long Integer(number=w406) -> (32bit integer=w411:i32)
                n219 = Build Array(w411) -> (w410:i32[])
                n220 = Select(t="3: The system is in a fault state", s=w414, f=w412) -> (s? t:f=w407:string)
                n221 = Format Into String(format string="%s.  Instr State = %s.", w407, w406) -> (resulting string=w404:string)  [unwired: 2 in, 1 out]
                n222 = Bundle By Name(cluster=w422, "Rt Loop Events"=RT_Loop_Events."Send Reply", "Info"=w404, "Data Array"=w410) -> (w421:T12)
              }
              frame "GT" {
                # "Get a Calibration/Resolution Table"
                n223 = Decimal String To Number(string=w425) -> (number=w424:i32)  [unwired: 3 out]
                n224 = case shown="0, Default" w424 {
                  tunnel: [w430 w431 w432 w433 w434 w435 w436 w437 w438 w439 w440 w441 w442 w443 w444 w445] -> w423
                  frame 0, Default {
                    n225 = global read "_RT Global.vi" "Q1 Cal"() -> (w430:dbl[][])
                  }
                  frame 1 {
                    n226 = global read "_RT Global.vi" "Q2 Cal"() -> (w431:dbl[][])
                  }
                  frame 2 {
                    n227 = global read "_RT Global.vi" "Q1 -Cal"() -> (w432:dbl[][])
                  }
                  frame 3 {
                    n228 = global read "_RT Global.vi" "Q2 -Cal"() -> (w433:dbl[][])
                  }
                  frame 4 {
                    n229 = global read "_RT Global.vi" "Q1 Res Hi"() -> (w434:dbl[][])
                  }
                  frame 5 {
                    n230 = global read "_RT Global.vi" "Q2 Res Hi"() -> (w435:dbl[][])
                  }
                  frame 6 {
                    n231 = global read "_RT Global.vi" "Q1 Res Med"() -> (w436:dbl[][])
                  }
                  frame 7 {
                    n232 = global read "_RT Global.vi" "Q2 Res Med"() -> (w437:dbl[][])
                  }
                  frame 8 {
                    n233 = global read "_RT Global.vi" "Q1 Res Lo"() -> (w438:dbl[][])
                  }
                  frame 9 {
                    n234 = global read "_RT Global.vi" "Q2 Res Lo"() -> (w439:dbl[][])
                  }
                  frame 10 {
                    n235 = global read "_RT Global.vi" "Q1 -Res Hi"() -> (w440:dbl[][])
                  }
                  frame 11 {
                    n236 = global read "_RT Global.vi" "Q2 -Res Hi"() -> (w441:dbl[][])
                  }
                  frame 12 {
                    n237 = global read "_RT Global.vi" "Q1 -Res Med"() -> (w442:dbl[][])
                  }
                  frame 13 {
                    n238 = global read "_RT Global.vi" "Q2 -Res Med"() -> (w443:dbl[][])
                  }
                  frame 14 {
                    n239 = global read "_RT Global.vi" "Q1 -Res Lo"() -> (w444:dbl[][])
                  }
                  frame 15 {
                    n240 = global read "_RT Global.vi" "Q2 -Res Lo"() -> (w445:dbl[][])
                  }
                }
                n241 = Flatten To String(anything=w423) -> (data string=w426:string)  [unwired: 1 in, 4 out]
                n242 = Bundle By Name(cluster=w429, "Rt Loop Events"=RT_Loop_Events."Send Reply", "Info"=w426) -> (w428:T12)
              }
              frame "IE" {
                # "Set Igore Lost Communication Error Flag\n0 = false\n1 = true (ignore error)"
                n243 = call <vilib>:"Trim Whitespace.vi"("string"=w449) -> ("trimmed string"=w448:string)  [unwired: 1 in]
                n244 = Not Equal?(x=w448, y="0") -> (x != y?=w446:bool)
                n245 = global write "_RT Global.vi" "IgnoreError"(w446) -> ()
                n246 = Bundle By Name(cluster=w452, "Rt Loop Events"=RT_Loop_Events."Send Reply") -> (w451:T12)
              }
              frame "MM" {
                # "Set Maximum Mass"
                n247 = global read "_RT Global.vi" "Max Mass"() -> (w457:dbl)
                n248 = Unflatten From String(type=w457, binary string=w458) -> (error out=w453:errorcluster)  [unwired: 1 in, 4 out]
                n249 = Bundle By Name(cluster=w455, "Rt Loop Events"=RT_Loop_Events."Send Reply", "error"=w453) -> (w454:T12)
              }
              frame "OG" {
                # "Get Startup Options"
                n250 = global read "_RT Global.vi" "StartupOptions"() -> (w460:T18)
                n251 = Flatten To String(anything=w460) -> (data string=w459:string)  [unwired: 1 in, 4 out]
                n252 = Bundle By Name(cluster=w462, "Rt Loop Events"=RT_Loop_Events."Send Reply", "Info"=w459) -> (w461:T12)
              }
              frame "OS" {
                # "Set Startup Options"
                n253 = global read "_RT Global.vi" "StartupOptions"() -> (w472:T18)
                n254 = Unflatten From String(type=w472, binary string=w464) -> (value=w471:T18)  [unwired: 1 in, 4 out]
                n255 = global write "_RT Global.vi" "StartupOptions"(w471) -> ()
                n256 = call "_RT Open Preference File.vi"() -> ("error"=w470:errorcluster, "refnum"=w469:T17)  [unwired: 6 out]
                n257 = call-poly <vilib>:"Write Key.vi"("section"="RT", "error in (no error)"=w470, "value"=w464, "key"="SUOpt", "refnum"=w469) -> ("error out"=w465:errorcluster, "refnum out"=w466:T17)  [unwired: 1 in, 4 out]
                n258 = call <vilib>:"Close Config Data.vi"("error in (no error)"=w465, "refnum"=w466) -> ()  [unwired: 1 in, 9 out]
                n259 = Bundle By Name(cluster=w474, "Rt Loop Events"=RT_Loop_Events."Send Reply") -> (w473:T12)
              }
              frame "P1" {
                # "Set COR POL, CUR POL for Latch2"
                n260 = Type Cast(type=u16 0, x=w482) -> (*(type *) &x=w476:u16)
                n261 = call "_FPGA Set Digi Line.vi"("States"=w476, "Line (Set Latch1)"=_RW_Status."Set Latch2" ("Write Mode (Do Write)")) -> ("error out"=w477:errorcluster)  [unwired: 2 in, 3 out]
                n262 = Bundle By Name(cluster=w479, "Rt Loop Events"=RT_Loop_Events."Send Reply", "error"=w477) -> (w478:T12)
              }
              frame "P2" {
                # "Set S1 POL, S2 POL for Latch3"
                n263 = Type Cast(type=u16 0, x=w490) -> (*(type *) &x=w484:u16)
                n264 = call "_FPGA Set Digi Line.vi"("States"=w484, "Line (Set Latch1)"=_RW_Status."Set Latch3" ("Write Mode (Do Write)")) -> ("error out"=w485:errorcluster)  [unwired: 2 in, 3 out]
                n265 = Bundle By Name(cluster=w487, "Rt Loop Events"=RT_Loop_Events."Send Reply", "error"=w485) -> (w486:T12)
              }
              frame "P3" {
                # "Set CEM POL for Latch4"
                n266 = Type Cast(type=u16 0, x=w498) -> (*(type *) &x=w492:u16)
                n267 = call "_FPGA Set Digi Line.vi"("States"=w492, "Line (Set Latch1)"=_RW_Status."Set Latch4" ("Write Mode (Do Write)")) -> ("error out"=w493:errorcluster)  [unwired: 2 in, 3 out]
                n268 = Bundle By Name(cluster=w495, "Rt Loop Events"=RT_Loop_Events."Send Reply", "error"=w493) -> (w494:T12)
              }
              frame "RA" {
                # "Read ADC"
                n269 = call "_FPGA Read ADC.vi"() -> ("error out"=w502:errorcluster, "Running"=w500:bool, "ADC Values"=w501:i32[])  [unwired: 3 in, 4 out]
                n270 = local write "Running"(w500) -> ()
                n271 = Bundle By Name(cluster=w505, "Rt Loop Events"=RT_Loop_Events."Send Reply", "Data Array"=w501, "error"=w502) -> (w504:T12)
              }
              frame "RP" {
                # "Toggle Roughing Pump"
                n272 = Not Equal?(x=w507, y="0") -> (x != y?=w508:bool)
                n273 = Boolean To (0,1)(Boolean=w508) -> (0, 1=w506:i16)
                n274 = call "_FPGA Set Digi Line.vi"("States"=w506, "Line (Set Latch1)"=_RW_Status."RP ON" ("Write Mode (Do Write)")) -> ("error out"=w510:errorcluster)  [unwired: 2 in, 3 out]
                n275 = Bundle By Name(cluster=w512, "Rt Loop Events"=RT_Loop_Events."Send Reply", "error"=w510) -> (w511:T12)
              }
              frame "RS" {
                w528 = u8 0 ("default (0 I32)")
                # "Toggle the startup/shut down"
                n276 = call <vilib>:"Trim Whitespace.vi"("string"=w531) -> ("trimmed string"=w530:string)  [unwired: 1 in]
                n277 = global read "_RT Global.vi" "InstrState"() -> (w517:T2)
                n278 = Decimal String To Number(string=w530, default (0L)=w528) -> (number=w529:u8)  [unwired: 2 out]
                n279 = In Range and Coerce(upper limit=u8 2, x=w529, lower limit=w528) -> (coerced(x)=w521:u8)  [unwired: 1 out]
                n280 = Not Equal?(x=w517, y=_RT_Instrument_State."Starting Up") -> (x != y?=w523:bool)
                n281 = Not Equal?(x=w517, y=_RT_Instrument_State."Turbo Startup") -> (x != y?=w518:bool)
                n282 = Not Equal?(x=w517, y=_RT_Instrument_State."Shutting Down") -> (x != y?=w515:bool)
                n283 = Not Equal?(x=w521, y=u8 1) -> (x != y?=w522:bool)
                n284 = Compound Arithmetic op=AND(w523, w518, w515) -> (w519:bool)
                n285 = Or(x=w522, y=w519) -> (x .or. y?=w520:bool)
                n286 = case shown="True" w520 {
                  tunnel: w521 -> [_ w536]
                  frame False {
                  }
                  frame True {
                    n287 = Greater Than 0?(x=w536) -> (x > 0?=w535:bool)
                    n288 = global write "_RT Global.vi" "StartupMode"(w536) -> ()
                    n289 = case shown="True" w535 {
                      frame False {
                      }
                      frame True {
                        n290 = call "_FPGA Turn LC Pump Off.vi"() -> ()  [unwired: 2 in]
                      }
                    }
                  }
                }
                n291 = Bundle By Name(cluster=w534, "Rt Loop Events"=RT_Loop_Events."Send Reply") -> (w533:T12)
              }
              frame "RU" {
                w538 = T4[] []  # Parameters
                # "Do a Run-Time Update"
                n292 = xnode "Read/Write Control"("FPGA VI Reference In"=w542) -> ("error out"=w541:errorcluster, "Running"=w537:bool)  [unwired: 1 in, 1 out]
                n293 = Unflatten From String(type=w538, binary string=w546) -> (value=w540:T4[])  [unwired: 1 in, 4 out]
                n294 = local write "Running"(w537) -> ()
                n295 = case shown="True" w537 {
                  tunnel: w541 -> [w547 w550]
                  tunnel: w540 -> [_ w548]
                  tunnel: [w547 w549] -> w539
                  frame False {
                  }
                  frame True {
                    n296 = call "_FPGA Runtime Update.vi"("error in"=w550, "Parameters"=w548) -> ("error out"=w549:errorcluster)  [unwired: 1 in, 4 out]
                  }
                }
                n297 = Bundle By Name(cluster=w544, "Rt Loop Events"=RT_Loop_Events."Send Reply", "error"=w539) -> (w543:T12)
              }
              frame "RV" {
                # "Read VAC Gauge"
                n298 = call "_FPGA Read Data.vi"("Read Mode (Do Read)"=_RW_Status."Read VAC" ("R/W Status")) -> ("error out"=w551:errorcluster, "Data"=w552:u32)  [unwired: 4 in, 1 out]
                n299 = Build Array(w552) -> (w554:u32[])
                n300 = Bundle By Name(cluster=w556, "Rt Loop Events"=RT_Loop_Events."Send Reply", "Data Array"=w554, "error"=w551) -> (w555:T12)
              }
              frame "SC" {
                # "Set Configuration"
                n301 = global read "_RT Global.vi" "Configuration 2"() -> (w574:T10)
                n302 = Unflatten From String(type=w574, binary string=w575) -> (value=w565:T10, error out=w568:errorcluster)  [unwired: 1 in, 3 out]
                n303 = Unbundle By Name(w565) -> ("Instrument"=w567:string[])
                n304 = Index Array(array=w567, index=2) -> (element=w561:string)
                n305 = call "_Get Startup File.vi"("FileName"="Config" ("key")) -> ("FilePath"=w559:path)
                n306 = Match Pattern(string=w561, regular expression="Simulation") -> (offset past match=w564:i32)  [unwired: 4 out]
                n307 = call "_Convert Model Name.vi"("Model"=w561) -> ("SingleSource"=w560:bool)  [unwired: 1 in, 1 out]
                n308 = global write "_RT Global.vi" "Configuration 2"(w565) -> ()
                n309 = Greater Or Equal To 0?(x=w564) -> (x >= 0?=w562:bool)
                n310 = Write to Binary File(file (use dialog)=w559, data=w565, error in=w568) -> (refnum out=w569:refnum<file>, error out=w570:errorcluster)  [unwired: 4 out]
                n311 = global write "_RT Global.vi" "Single Source"(w560) -> ()
                n312 = global write "_RT Global.vi" "Simulation"(w562) -> ()
                n313 = Close File(refnum=w569, error in=w570) -> ()  [unwired: 2 out]
                n314 = Bundle By Name(cluster=w572, "Rt Loop Events"=RT_Loop_Events."Send Reply") -> (w571:T12)
              }
              frame "SL" {
                # "Set LC Outputs"
                n315 = Type Cast(type=u16 0, x=w578) -> (*(type *) &x=w577:u16)
                n316 = call "_FPGA Write Data.vi"("Write Mode (Do Write)"=_RW_Status."Set LC Out", "Address"=w577) -> ("error out"=w576:errorcluster)  [unwired: 4 in, 2 out]
                n317 = Bundle By Name(cluster=w582, "Rt Loop Events"=RT_Loop_Events."Send Reply", "error"=w576) -> (w581:T12)
              }
              frame "SO" {
                # "Set Oscillator"
                n318 = Unflatten From String(type=u32[] [], binary string=w588) -> (value=w591:u32[])  [unwired: 1 in, 4 out]
                n319 = xnode "Read/Write Control"("FPGA VI Reference In"=w593) -> ("error out"=w592:errorcluster, "Running"=w587:bool)  [unwired: 1 in, 1 out]
                n320 = local write "Running"(w587) -> ()
                n321 = Index Array(array=w591) -> (element #1=w586:u32, element #2=w585:u32, element #3=w584:u32)  [unwired: 3 in]
                n322 = call "_FPGA Set Oscillator.vi"("Param 3"=w584, "error in"=w592, "Param 2"=w585, "Param 1"=w586) -> ("error out"=w590:errorcluster)  [unwired: 1 in, 3 out]
                n323 = Bundle By Name(cluster=w595, "Rt Loop Events"=RT_Loop_Events."Send Reply", "error"=w590) -> (w594:T12)
              }
              frame "SP" {
                # "Set PIC"
                n324 = Unflatten From String(type=u32[] [], binary string=w608) -> (value=w602:u32[])  [unwired: 1 in, 4 out]
                n325 = xnode "Read/Write Control"("FPGA VI Reference In"=w604) -> ("error out"=w603:errorcluster, "Running"=w600:bool)  [unwired: 1 in, 1 out]
                n326 = local write "Running"(w600) -> ()
                n327 = case shown="False" w600 {
                  tunnel: w603 -> [w614 w616]
                  tunnel: w602 -> [w612 _]
                  tunnel: [w613 w615] -> w599
                  tunnel: [w609 _] -> w598
                  frame False {
                    n328 = Index Array(array=w612) -> (element #1=w611:u32, element #2=w610:u32)  [unwired: 2 in]
                    n329 = call "_FPGA Set PIC.vi"("error in"=w614, "Param 2"=w610, "Param 1"=w611) -> ("error out"=w613:errorcluster, "Data"=w609:u32)  [unwired: 2 in, 1 out]
                  }
                  frame True {
                    n330 = call "_Construct Error Cluster.vi"("error in"=w616, "reason"="Cannot send command to PIC because the instrument is busy.") -> ("error out"=w615:errorcluster)  [unwired: 2 in, 3 out]
                  }
                }
                n331 = Build Array(w598) -> (w597:u32[])
                n332 = Bundle By Name(cluster=w606, "Rt Loop Events"=RT_Loop_Events."Send Reply", "Data Array"=w597, "error"=w599) -> (w605:T12)
              }
              frame "SS" {
                # "Send Serial Command"
                n333 = Unflatten From String(type=T15 {"Port Type"=0, "baud rate (9600)"=9600, "data bits (8)"=8, "stop bits (1)"=10, "parity (0:none)"=0, "DoRead"=FALSE, "Command"=""} ("Serial Command"), binary string=w628) -> (value=w622:T15)  [unwired: 1 in, 4 out]
                n334 = xnode "Read/Write Control"("FPGA VI Reference In"=w624) -> ("error out"=w623:errorcluster, "Running"=w621:bool)  [unwired: 1 in, 1 out]
                n335 = local write "Running"(w621) -> ()
                n336 = case shown="False" w621 {
                  tunnel: w623 -> [w631 w634]
                  tunnel: w622 -> [w630 _]
                  tunnel: [w632 w633] -> w620
                  tunnel: [w629 _] -> w618
                  frame False {
                    n337 = call "_FPGA Send Serial.vi"("error in"=w631, "Serial Command"=w630) -> ("error out"=w632:errorcluster, "Reply"=w629:string)  [unwired: 2 in, 2 out]
                  }
                  frame True {
                    n338 = call "_Construct Error Cluster.vi"("error in"=w634, "reason"="Cannot send command to serial port because the instrument is busy.") -> ("error out"=w633:errorcluster)  [unwired: 2 in, 3 out]
                  }
                }
                n339 = Bundle By Name(cluster=w626, "Rt Loop Events"=RT_Loop_Events."Send Reply", "Info"=w618, "error"=w620) -> (w625:T12)
              }
              frame "ST" {
                # "Start a Run"
                n340 = global read "_RT Global.vi" "FPGA semaphore"() -> (w638:T9)
                n341 = Unbundle By Name(w641) -> ("Parameter"=w643:T3)
                n342 = Unflatten From String(type=w643, binary string=w644) -> (value=w636:T3)  [unwired: 1 in, 4 out]
                n343 = stacked-sequence {
                  tunnel: w637 -> [_ w652 _ _]
                  tunnel: w636 -> [_ w653 _ _]
                  tunnel: [_ w658 _ _] -> w639
                  tunnel: w638 -> [w651 _ _ w675]
                  frame #0 {
                    n344 = call <vilib>:"Acquire Semaphore.vi"("ms timeout (-1)"=2000, "semaphore"=w651) -> ("timed out"=w645:bool)  [unwired: 1 in, 4 out]
                    n345 = local read "Running"() -> (w648:bool)
                    n346 = global read "_RT Global.vi" "InstrState"() -> (w649:T2)
                    n347 = Format Into String(format string="Start Run: Instr State = %s; FPGA Running = %s;  Time Out = %s.", w649, w648, w645) -> (resulting string=w646:string)  [unwired: 2 in, 1 out]
                    n348 = call "_RT Event.vi"("Event"=w646) -> ()  [unwired: 2 in, 5 out]
                  }
                  frame #1 {
                    n349 = call "_Update Parameter Data.vi"("Parameter"=w653) -> ("error out"=w654:errorcluster, "RF Only"=w655:bool)  [unwired: 2 in, 3 out]
                    n350 = local read "Ready"() -> (w656:bool)
                    n351 = Or(x=w655, y=w656) -> (x .or. y?=w657:bool)
                    n352 = case shown="True" w657 {
                      tunnel: w652 -> [_ w666]
                      tunnel: w653 -> [_ w668]
                      tunnel: [w660 w665] -> w658
                      tunnel: w654 -> [_ w662]
                      frame False {
                        n353 = call "_Construct Error Cluster.vi"("reason"="8016: A run is in progress or system is not ready.", "errorCode"=8016) -> ("error out"=w660:errorcluster)  [unwired: 2 in, 3 out]
                      }
                      frame True {
                        n354 = Unbundle By Name(w668) -> ("RunMode"=w663:i32)
                        "RunMode" <- w663
                        n355 = case shown="3, 6, 7" w663 {
                          tunnel: w662 -> [w669 w670]
                          tunnel: [w669 w670] -> w667
                          frame 0, Default {
                          }
                          frame 3, 6, 7 {
                            n356 = call "_FPGA Read Counter.vi"() -> ()  [unwired: 2 in, 4 out]
                          }
                        }
                        n357 = case shown="No Error" w667 {
                          selector: w667 -> [_ w673]
                          tunnel: w666 -> [w672 _]
                          tunnel: [_ w673] -> w665
                          tunnel: [w671 _] -> w664
                          frame No Error {
                            w671 = TRUE ("Start")
                            n358 = xnode "Read/Write Control"("FPGA VI Reference In"=w672, "Start"=w671) -> ()  [unwired: 1 in, 2 out]
                          }
                          frame Error {
                          }
                        }
                        "Running" <- w664
                      }
                    }
                  }
                  frame #2 {
                    n359 = Wait (ms)(milliseconds to wait=u32 180) -> ()  [unwired: 1 out]
                  }
                  frame #3 {
                    n360 = call <vilib>:"Release Semaphore.vi"("semaphore"=w675) -> ()  [unwired: 1 in, 6 out]
                  }
                }
                n361 = Bundle By Name(cluster=w641, "Rt Loop Events"=RT_Loop_Events."Send Reply", "Parameter"=w636, "error"=w639) -> (w640:T12)
              }
              frame "TT" {
                w686 = u16 405 ("Address")
                # "Run Table Test"
                n362 = Unflatten From String(type=u32[] [], binary string=w691) -> (value=w689:u32[])  [unwired: 1 in, 4 out]
                n363 = Index Array(array=w689) -> (element #1=w688:u32, element #2=w685:u32)  [unwired: 2 in]
                n364 = Increment(x=w686) -> (x+1=w683:u16)
                n365 = call "_FPGA Write Data.vi"("Data"=w688, "Address"=w686) -> ("error out"=w687:errorcluster)  [unwired: 4 in, 2 out]
                n366 = call "_FPGA Write Data.vi"("error in"=w687, "Data"=w685, "Address"=w683) -> ("error out"=w684:errorcluster)  [unwired: 3 in, 2 out]
                n367 = xnode "Read/Write Control"("FPGA VI Reference In"=w690, "error in"=w684, "R/W Status"=_RW_Status."Table Test") -> ("FPGA VI Reference Out"=w695:refnum<k20>, "error out"=w694:errorcluster)
                n368 = xnode "Read/Write Control"("FPGA VI Reference In"=w695, "error in"=w694, "Read/Write"=TRUE ("Data Written")) -> ("error out"=w696:errorcluster)  [unwired: 1 out]
                n369 = call "_FPGA Wait Done.vi"("error in"=w696, "Indicator"=_FPGA_Indicator."Done") -> ("error out"=w682:errorcluster)  [unwired: 3 in, 2 out]
                n370 = Increment(x=w683) -> (x+1=w679:u16)
                n371 = call "_FPGA Read Data.vi"("error in"=w682, "Address"=w679) -> ("error out"=w681:errorcluster, "Data"=w677:u32)  [unwired: 3 in, 1 out]
                n372 = Increment(x=w679) -> (x+1=w680:u16)
                n373 = call "_FPGA Read Data.vi"("error in"=w681, "Address"=w680) -> ("error out"=w678:errorcluster, "Data"=w676:u32)  [unwired: 3 in, 1 out]
                n374 = Build Array(w677, w676) -> (w693:u32[])
                n375 = Bundle By Name(cluster=w701, "Rt Loop Events"=RT_Loop_Events."Send Reply", "Data Array"=w693, "error"=w678) -> (w700:T12)
              }
              frame "UT" {
                # "Update a Calibration/Resolution Table"
                n376 = Unflatten From String(type=cluster{"Type":u16, "Table":dbl[][]} {"Type"=0, "Table"=[]} ("Calibration"), binary string=w705) -> (value=w706:cluster{"Type":u16, "Table":dbl[][]})  [unwired: 1 in, 4 out]
                n377 = Unbundle By Name(w706) -> ("Type"=w704:u16, "Table"=w703:dbl[][])
                n378 = stacked-sequence {
                  tunnel: [_ w748] -> w709
                  tunnel: w704 -> [w714 w747]
                  tunnel: w703 -> [w712 _]
                  frame #0 {
                    n379 = case shown="0, Default" w714 {
                      tunnel: ["Cal" ("key") "Cal2" ("key") "Cal3" ("key") "Cal4" ("key") "Res" ("key") "Res2" ("key") "Res3" ("key") "Res4" ("key") "Res5" ("key") "Res6" ("key") "Res7" ("key") "Res8" ("key") "Res9" ("key") "Res10" ("key") "Res11" ("key") "Res12" ("key")] -> w713
                      frame 0, Default {
                      }
                      frame 1 {
                      }
                      frame 2 {
                      }
                      frame 3 {
                      }
                      frame 4 {
                      }
                      frame 5 {
                      }
                      frame 6 {
                      }
                      frame 7 {
                      }
                      frame 8 {
                      }
                      frame 9 {
                      }
                      frame 10 {
                      }
                      frame 11 {
                      }
                      frame 12 {
                      }
                      frame 13 {
                      }
                      frame 14 {
                      }
                      frame 15 {
                      }
                    }
                    n380 = case shown="3" w714 {
                      tunnel: w712 -> [w715 w716 w717 w718 w719 w720 w721 w722 w723 w724 w725 w726 w727 w728 w729 w730]
                      frame 0, Default {
                        n381 = global write "_RT Global.vi" "Q1 Cal"(w715) -> ()
                      }
                      frame 1 {
                        n382 = global write "_RT Global.vi" "Q2 Cal"(w716) -> ()
                      }
                      frame 2 {
                        n383 = global write "_RT Global.vi" "Q1 -Cal"(w717) -> ()
                      }
                      frame 3 {
                        n384 = global write "_RT Global.vi" "Q2 -Cal"(w718) -> ()
                      }
                      frame 4 {
                        n385 = global write "_RT Global.vi" "Q1 Res Hi"(w719) -> ()
                      }
                      frame 5 {
                        n386 = global write "_RT Global.vi" "Q2 Res Hi"(w720) -> ()
                      }
                      frame 6 {
                        n387 = global write "_RT Global.vi" "Q1 Res Med"(w721) -> ()
                      }
                      frame 7 {
                        n388 = global write "_RT Global.vi" "Q2 Res Med"(w722) -> ()
                      }
                      frame 8 {
                        n389 = global write "_RT Global.vi" "Q1 Res Lo"(w723) -> ()
                      }
                      frame 9 {
                        n390 = global write "_RT Global.vi" "Q2 Res Lo"(w724) -> ()
                      }
                      frame 10 {
                        n391 = global write "_RT Global.vi" "Q1 -Res Hi"(w725) -> ()
                      }
                      frame 11 {
                        n392 = global write "_RT Global.vi" "Q2 -Res Hi"(w726) -> ()
                      }
                      frame 12 {
                        n393 = global write "_RT Global.vi" "Q1 -Res Med"(w727) -> ()
                      }
                      frame 13 {
                        n394 = global write "_RT Global.vi" "Q2 -Res Med"(w728) -> ()
                      }
                      frame 14 {
                        n395 = global write "_RT Global.vi" "Q1 -Res Lo"(w729) -> ()
                      }
                      frame 15 {
                        n396 = global write "_RT Global.vi" "Q2 -Res Lo"(w730) -> ()
                      }
                    }
                    n397 = call "_Save RT Table.vi"("Table"=w712, "key"=w713) -> ()  [unwired: 1 in, 5 out]
                  }
                  frame #1 {
                    n398 = call "_Update Cal or Res Data.vi"("Table Type"=w747) -> ("error out"=w748:errorcluster)  [unwired: 2 in, 4 out]
                  }
                }
                n399 = Bundle By Name(cluster=w711, "Rt Loop Events"=RT_Loop_Events."Send Reply", "error"=w709) -> (w708:T12)
              }
              frame Default {
                n400 = Format Into String(format string="Message Type: %s, not recognized by firmware command receiver.", w755) -> (resulting string=w753:string)  [unwired: 2 in, 1 out]
                n401 = call "_Construct Error Cluster.vi"("reason"=w753) -> ("error out"=w749:errorcluster)  [unwired: 3 in, 3 out]
                n402 = Bundle By Name(cluster=w751, "Rt Loop Events"=RT_Loop_Events."Send Reply", "error"=w749) -> (w750:T12)
              }
            }
            n403 = local write "Disconnection#"(u8 0 ("Disconnection#")) -> ()
          }
          frame True {
            # "No command received from the host at this time,\nor the host has been disconnected."
            n404 = local read "Disconnection#"() -> (w760:u8)
            n405 = Greater?(x=w760, y=u8 2) -> (0:w757:bool)
            n406 = Wait Until Next ms Multiple(millisecond multiple=u32 380 ("milliseconds to wait")) -> ()  [unwired: 1 out]
            n407 = case shown="True" w757 {
              tunnel: w760 -> [w766 _]
              tunnel: w759 -> [_ w769]
              tunnel: [RT_Loop_Events."Wait for Command" ("Rt Loop Events") RT_Loop_Events."Wait for Connection" ("Rt Loop Events")] -> w758
              frame False {
                n408 = Increment(x=w766) -> (x+1=→"Disconnection#":u8)
              }
              frame True {
                n409 = TCP Close Connection(connection ID=w769, abort (F)=TRUE) -> ()  [unwired: 1 in, 2 out]
                "Connected?" <- FALSE ("Connected?")
              }
            }
            n410 = Bundle By Name(cluster=w763, "Rt Loop Events"=w758) -> (w762:T12)
          }
        }
      }
      frame "Send Reply" {
        w775 = i32[] []  # Data Array
        w773 = errorcluster {"status"=FALSE, "code"=0, "source"=""}  # error
        w776 = ""  # Info
        # "Send a reply back to the host after receiving each command"
        n411 = Unbundle By Name(w778) -> ("Connection ID"=w780:refnum<k5>, "Info"=w781:string, "Data Array"=w784:i32[], "error"=w774:errorcluster)
        n412 = Bundle("Info"=w781, "Data Array"=w784, "error"=w774) -> (w772:T19)  [unwired: 1 out]
        n413 = Flatten To String(anything=w772) -> (data string=w782:string)  [unwired: 1 in, 4 out]
        n414 = call "_TCP Msg Write.vi"("Data Stream"=w782, "Message Type"="RE" ("Name"), "connection ID"=w780) -> ()  [unwired: 2 in, 7 out]
        n415 = Bundle By Name(cluster=w778, "Rt Loop Events"=RT_Loop_Events."Wait for Command", "Info"=w776, "Data Array"=w775, "error"=w773) -> (w777:T12)
      }
    }
  }
  n416 = Decimal String To Number(string=w30, default (0L)=0 ("default (0 I32)")) -> (number=w29:i32)  [unwired: 2 out]
  n417 = Greater Or Equal To 0?(x=w19) -> (x >= 0?=w17:bool)
  n418 = Greater Or Equal To 0?(x=w9) -> (x >= 0?=w3:bool)
  n419 = Or(x=w3, y=w2) -> (x .or. y?=w1:bool)
  n420 = call "_Convert Model Name.vi"("Model"=w8) -> ("SingleSource"=w16:bool)  [unwired: 1 in, 1 out]
  n421 = Greater Than 0?(x=w29) -> (x > 0?=w28:bool)
  n422 = case shown="True" w28 {
    tunnel: [_RT_Instrument_State."Initializing" ("InstrState") _RT_Instrument_State."Starting Up" ("InstrState")] -> w38
    frame False {
    }
    frame True {
      n423 = global write "_RT Global.vi" "StartupMode"(u8 0 ("StartupMode")) -> ()
    }
  }
  n424 = global write "_RT Global.vi" "UseLeybold"(w1) -> ()
  n425 = global write "_RT Global.vi" "Simulation"(w17) -> ()
  n426 = global write "_RT Global.vi" "Single Source"(w16) -> ()
  n427 = while {
    tunnel: w15 -> [w788]
    shift-right: [w792] -> _
    shift-left: w38 -> [w791]
    i -> [w790]
    stop <- FALSE stop-if-true
    n428 = case shown="\"Turbo Startup\"" w791 {
      selector: w791 -> [_ w811 _ _ w833 _ _ _ w861 _ w886 w903 _ _ w994 w1021 w1040 w1073 _ _]
      tunnel: w788 -> [_ _ _ _ _ _ _ _ _ _ _ _ w922 _ _ _ _ _ _ _]
      tunnel: [_RT_Instrument_State."Mass Spectrometer is Off" ("InstrState") w810 w815 _RT_Instrument_State."Roughing Pump Ready" ("InstrState") w834 w845 _RT_Instrument_State."Initializing" ("t") _RT_Instrument_State."Going to Standby" ("t") w860 _RT_Instrument_State."24V Standby" ("InstrState") w885 w902 w923 _RT_Instrument_State."Ready" ("InstrState") w996 w1022 w1043 w1070 w1084 _RT_Instrument_State."Shutting Down" ("t")] -> w792
      tunnel: w790 -> [_ _ _ _ _ _ _ _ _ _ _ _ _ _ w989 _ w1038 _ _ _]
      frame "Initializing" {
        w796 = T22 11 items=["Same", "Empty", "VacFail", "Cancel", "CheckGas", "EleFail", "Probe1Fail", "Probe2Fail", "HeaterFail", "DoorOpen", "CheckComm", "PressStart"] ("Line2Msg (same)")
        w797 = T23 2 items=["Same", "Empty", "Connected", "Starting", "Stopping", "Action", "On", "Service", "Call", "Acquiring", "Source"] ("Line1Msg (same)")
        w799 = FALSE ("Connected?")
        # "Going to System Off State"
        n429 = call "_FPGA Set LEDs.vi"("LED Command"=_LED_States."Off BRP") -> ("error out"=w801:errorcluster)  [unwired: 3 in, 3 out]
        n430 = Wait (ms)(milliseconds to wait=u32 1800) -> ()  [unwired: 1 out]
        n431 = call "_FPGA Set LCD Msg.vi"("error in"=w801, "Line2Msg (same)"=w796, "Line1Msg (same)"=w797) -> ("error out"=w794:errorcluster)  [unwired: 4 in, 2 out]
        n432 = call "_FPGA Send LCD.vi"("error in (no error)"=w794, "Command"=_RT_LED_Num."ReadKey" ("LED#")) -> ()  [unwired: 2 in, 5 out]
        n433 = global write "_RT Global.vi" "StartupMode"(u8 2 ("StartupMode")) -> ()
        n434 = local write "Running"(FALSE ("Connected?")) -> ()
        n435 = call "_RT Event.vi"("Event"="Mass Spectrometer is OFF. Power Connected") -> ()  [unwired: 2 in, 5 out]
        "Ready" <- w799
        "Fault" <- w799
      }
      frame "Mass Spectrometer is Off" {
        # "Wait for the start up command"
        n436 = call "_FPGA Read Key.vi"("CurStartupMode (0)"=u8 2, "ForStart (F)"=TRUE) -> ("Key Pressed"=w808:bool)  [unwired: 3 in, 3 out]
        n437 = Select(t=_RT_Instrument_State."Starting Up", s=w808, f=w811) -> (s? t:f=w810:T2)
      }
      frame "Starting Up" {
        w813 = FALSE ("Status LED")
        # "Start a startup sequence"
        n438 = call "_FPGA Send LCD.vi"("Command"=_RT_LED_Num."ReadKey" ("LED#")) -> ("error out"=w812:errorcluster)  [unwired: 4 in, 3 out]
        n439 = call "_Update Start Up.vi"("error in (no error)"=w812) -> ("Next InstrState"=w815:T2)  [unwired: 2 in, 4 out]
        n440 = local write "Ready"(w813) -> ()
        n441 = local write "Fault"(w813) -> ()
      }
      frame "Going to Standby" {
        w819 = T23 8 items=["Same", "Empty", "Connected", "Starting", "Stopping", "Action", "On", "Service", "Call", "Acquiring", "Source"] ("Line1Msg (same)")
        n442 = call "_FPGA Read ADC.vi"() -> ("error out"=w816:errorcluster)  [unwired: 3 in, 6 out]
        n443 = call "_FPGA Check Source ID.vi"("error in (no error)"=w816) -> ("Source ID OK"=w821:bool)
        n444 = call "_FPGA Set Parameters.vi"("ExhaustGas (on)"=FALSE, "error in"=w816, "HSID Temp (on)"=w821) -> ("error out"=w823:errorcluster)  [unwired: 6 in, 2 out]
        n445 = call "_FPGA Set LEDs.vi"("error in (no error)"=w823, "LED Command"=_LED_States."Off BRP") -> ("error out"=w822:errorcluster)  [unwired: 2 in, 3 out]
        n446 = call "_FPGA Set LEDs.vi"("error in (no error)"=w822, "LED Command"=_LED_States."Solid P") -> ("error out"=w827:errorcluster)  [unwired: 2 in, 3 out]
        n447 = call "_FPGA Set LCD Msg.vi"("error in"=w827, "Line1Msg (same)"=w819) -> ("error out"=w828:errorcluster)  [unwired: 5 in, 2 out]
        n448 = call "_RT Event.vi"("Event"="Roughing Pump Ready state.") -> ()  [unwired: 2 in, 5 out]
        n449 = call "_FPGA Send LCD.vi"("error in (no error)"=w828, "Command"=_RT_LED_Num."ReadKey" ("LED#")) -> ()  [unwired: 3 in, 4 out]
        n450 = global write "_RT Global.vi" "StartupMode"(u8 1 ("StartupMode")) -> ()
        n451 = local write "Ready"(FALSE ("Status LED")) -> ()
        n452 = local write "Fault"(TRUE ("Fault")) -> ()
      }
      frame "Roughing Pump Ready" {
        n453 = global read "_RT Global.vi" "StartupMode"() -> (w832:u8)
        n454 = case shown="1, Default" w832 {
          tunnel: [_RT_Instrument_State."Turbo Startup" ("InstrState") w838 _RT_Instrument_State."Shutting Down" ("InstrState")] -> w834
          tunnel: w833 -> [_ w836 _]
          frame 0 {
            # "Continue the startup sequence"
          }
          frame 1, Default {
            # "Wait for Start key to restart the system"
            n455 = call "_FPGA Read Key.vi"("CurStartupMode (0)"=u8 1, "ForStart (F)"=TRUE) -> ("Key Pressed"=w841:bool)  [unwired: 3 in, 3 out]
            n456 = Select(t=_RT_Instrument_State."Turbo Startup", s=w841, f=w836) -> (s? t:f=w838:T2)
          }
          frame 2 {
            # "Received a shutdown command"
          }
        }
      }
      frame "Turbo Startup" {
        # "Continue the startup sequence"
        n457 = call "_FPGA Send LCD.vi"("Command"=_RT_LED_Num."ReadKey" ("LED#")) -> ("error out"=w843:errorcluster)  [unwired: 4 in, 3 out]
        n458 = call "_Update Start Up Turbo.vi"("error in (no error)"=w843) -> ("Next InstrState"=w845:T2)  [unwired: 2 in, 4 out]
      }
      frame "Turning Power Off" {
        w846 = T23 4 items=["Same", "Empty", "Connected", "Starting", "Stopping", "Action", "On", "Service", "Call", "Acquiring", "Source"] ("Line1Msg (same)")
        n459 = call "_FPGA Set LCD Msg.vi"("Line1Msg (same)"=w846) -> ()  [unwired: 6 in, 3 out]
        n460 = local write "Ready"(FALSE ("Status LED")) -> ()
        n461 = local write "Fault"(TRUE ("Status LED")) -> ()
        n462 = Wait (ms)(milliseconds to wait=u32 1800) -> ()  [unwired: 1 out]
      }
      frame "Turning Turbo Off" {
        n463 = stacked-sequence {
          frame #0 {
            n464 = Wait (ms)(milliseconds to wait=u32 1800) -> ()  [unwired: 1 out]
          }
          frame #1 {
            n465 = call "_FPGA Send LCD.vi"("Command"=_RT_LED_Num."ReadKey" ("LED#")) -> ()  [unwired: 4 in, 4 out]
          }
        }
        n466 = local write "Ready"(FALSE ("Status LED")) -> ()
        n467 = local write "Fault"(TRUE ("Status LED")) -> ()
      }
      frame "Turbopump Ready" {
        w857 = T23 5 items=["Same", "Empty", "Connected", "Starting", "Stopping", "Action", "On", "Service", "Call", "Acquiring", "Source"] ("Line1Msg (same)")
        n468 = global read "_RT Global.vi" "StartupMode"() -> (w862:u8)
        n469 = local write "Fault"(TRUE ("Status LED")) -> ()
        n470 = call "_FPGA Set LCD Msg.vi"("Line1Msg (same)"=w857) -> ("error out"=w856:errorcluster)  [unwired: 6 in, 2 out]
        n471 = case shown="Default" w862 {
          tunnel: [w869 _RT_Instrument_State."Shutting Down" ("InstrState") _RT_Instrument_State."Checking Vacuum" ("InstrState")] -> w860
          tunnel: w861 -> [w866 _ _]
          tunnel: w856 -> [_ _ _]
          frame Default {
            # "Allow system to shut down from this state"
            n472 = local read "Connected?"() -> (w868:bool)
            n473 = call "_FPGA Read Key.vi"("CurStartupMode (0)"=u8 1) -> ("error out"=w863:errorcluster, "Key Pressed"=w871:bool)  [unwired: 4 in, 2 out]
            n474 = call "_FPGA System Polling.vi"("error in (no error)"=w863, "Connected?"=w868, "CurInstrState"=w866) -> ("Running"=w867:bool, "Next InstrState"=w865:T2)  [unwired: 2 in, 2 out]
            n475 = local write "Running"(w867) -> ()
            n476 = Select(t=_RT_Instrument_State."Shutting Down", s=w871, f=w865) -> (s? t:f=w869:T2)
          }
          frame 2 {
            # "Received a shutdown command"
          }
          frame 0 {
            # "Received a startup command"
          }
        }
        n477 = local write "Ready"(FALSE ("Status LED")) -> ()
      }
      frame "Go to 24V Standby" {
        w877 = T23 7 items=["Same", "Empty", "Connected", "Starting", "Stopping", "Action", "On", "Service", "Call", "Acquiring", "Source"] ("Line1Msg (same)")
        n478 = local write "Fault"(TRUE ("Status LED")) -> ()
        n479 = call "_FPGA Set LCD Msg.vi"("Line1Msg (same)"=w877) -> ("error out"=w874:errorcluster)  [unwired: 6 in, 2 out]
        n480 = global read "_RT Global.vi" "Ele On"() -> (w876:bool)
        n481 = local write "Ready"(FALSE ("Status LED")) -> ()
        n482 = case shown="True" w876 {
          tunnel: w874 -> [_ _]
          frame False {
          }
          frame True {
            # "Turn off electronics"
            n483 = call "_FPGA Toggle Electronics.vi"() -> ()  [unwired: 3 in, 6 out]
          }
        }
        n484 = call "_RT Event.vi"("Event"="Going to 24V Standby state.") -> ()  [unwired: 2 in, 5 out]
      }
      frame "Turbopump Ready-Waiting" {
        w882 = T23 8 items=["Same", "Empty", "Connected", "Starting", "Stopping", "Action", "On", "Service", "Call", "Acquiring", "Source"] ("Line1Msg (same)")
        n485 = global read "_RT Global.vi" "StartupMode"() -> (w887:u8)
        n486 = local write "Fault"(TRUE ("Status LED")) -> ()
        n487 = call "_FPGA Set LCD Msg.vi"("Line1Msg (same)"=w882) -> ("error out"=w881:errorcluster)  [unwired: 6 in, 2 out]
        n488 = case shown="Default" w887 {
          tunnel: [w892 _RT_Instrument_State."Shutting Down" ("InstrState") _RT_Instrument_State."Checking Vacuum" ("InstrState")] -> w885
          tunnel: w886 -> [w895 _ _]
          tunnel: w881 -> [_ _ _]
          frame Default {
            # "Allow system to proceed to ready from this state"
            n489 = local read "Connected?"() -> (w897:bool)
            n490 = call "_FPGA Read Key.vi"("CurStartupMode (0)"=u8 1, "ForStart (F)"=TRUE) -> ("error out"=w888:errorcluster, "Key Pressed"=w891:bool)  [unwired: 3 in, 2 out]
            n491 = call "_FPGA System Polling.vi"("error in (no error)"=w888, "Waiting (F)"=TRUE, "Connected?"=w897, "CurInstrState"=w895) -> ("Running"=w896:bool, "Next InstrState"=w890:T2)  [unwired: 1 in, 2 out]
            n492 = case shown="True" w891 {
              tunnel: [w898 _RT_Instrument_State."Checking Vacuum" ("t")] -> w892
              tunnel: w890 -> [w898 _]
              frame False {
              }
              frame True {
              }
            }
            n493 = local write "Running"(w896) -> ()
          }
          frame 2 {
            # "Received a shutdown command"
          }
          frame 0 {
            # "Received a startup command"
          }
        }
        n494 = local write "Ready"(FALSE ("Status LED")) -> ()
      }
      frame "24V Standby" {
        n495 = global read "_RT Global.vi" "StartupMode"() -> (w904:u8)
        n496 = case shown="Default" w904 {
          tunnel: [w912 _RT_Instrument_State."Shutting Down" ("InstrState") _RT_Instrument_State."Starting Up" ("InstrState")] -> w902
          tunnel: w903 -> [w910 _ _]
          frame Default {
            # "Allow system to restart from this state"
            n497 = local read "Connected?"() -> (w916:bool)
            n498 = call "_FPGA Read Key.vi"("CurStartupMode (0)"=u8 1, "ForStart (F)"=TRUE) -> ("error out"=w905:errorcluster, "Key Pressed"=w908:bool)  [unwired: 3 in, 2 out]
            n499 = call "_FPGA System Polling.vi"("error in (no error)"=w905, "Waiting (F)"=TRUE, "Connected?"=w916, "CurInstrState"=w910) -> ("Running"=w915:bool, "Next InstrState"=w911:T2)  [unwired: 1 in, 2 out]
            n500 = Not Equal?(x=w910, y=w911) -> (x != y?=w909:bool)
            n501 = Or(x=w908, y=w909) -> (x .or. y?=w907:bool)
            n502 = case shown="False" w907 {
              tunnel: [w917 _RT_Instrument_State."Starting Up" ("t")] -> w912
              tunnel: w911 -> [w917 _]
              frame False {
              }
              frame True {
                n503 = global write "_RT Global.vi" "StartupMode"(u8 0 ("StartupMode")) -> ()
              }
            }
            n504 = local write "Running"(w915) -> ()
          }
          frame 2 {
            # "Received a shutdown command"
          }
          frame 0 {
            # "Received a startup command"
          }
        }
      }
      frame "Checking Vacuum" {
        n505 = stacked-sequence {
          seq-local: [w927 _] -> [_ w946]
          seq-local: [w926 _] -> [_ w945]
          seq-local: [w925 _] -> [_ w944]
          tunnel: w922 -> [_ w947]
          tunnel: [_ w948] -> w923
          frame #0 {
            n506 = Tick Count (ms)() -> (millisecond timer value=w928:u32)
            n507 = call "_FPGA Set LEDs.vi"("LED Command"=_LED_States."Off BRP") -> ("error out"=w924:errorcluster)  [unwired: 3 in, 3 out]
            n508 = while {
              tunnel: w928 -> [w940]
              tunnel: [w939] -> w927
              tunnel: [w937] -> w926
              tunnel: [w930] -> w925
              tunnel: w924 -> [_]
              stop <- w932 stop-if-true
              w934 = u32 1800000  # 30min timeout
              n509 = Wait (ms)(milliseconds to wait=u32 800) -> (millisecond timer value=w942:u32)
              n510 = Subtract(x=w942, y=w940) -> (x-y=w935:u32)
              n511 = call "_Check Limit.vi"("Header"="Pumping 2:" ("Header (10Ch)"), "Current"=w935, "Max (100)"=w934) -> ("Max Reached"=w933:bool, "ProgressBar"=w931:string)  [unwired: 1 in, 2 out]
              n512 = call "_FPGA Check Vacuum.vi"() -> ("Vac OK"=w939:bool, "Source OK"=w937:bool, "Stop"=w938:bool, "Shutdown"=w930:bool)  [unwired: 2 out]
              n513 = Or(x=w938, y=w933) -> (x .or. y?=w932:bool)
              n514 = case shown="False" w932 {
                tunnel: w931 -> [w943 _]
                frame False {
                  n515 = call "_FPGA Set LCD Msg.vi"("Info"=w943) -> ()  [unwired: 6 in, 3 out]
                }
                frame True {
                }
              }
            }
          }
          frame #1 {
            n516 = case shown="True" w946 {
              tunnel: [w951 w966] -> w948
              tunnel: w947 -> [_ w960]
              tunnel: w945 -> [_ w961]
              tunnel: w944 -> [w949 _]
              frame False {
                # "User aborted vacuum check or 20min timeout:\nHigh vacuum not achieved."
                n517 = case shown="False" w949 {
                  tunnel: [_RT_Instrument_State."Turbopump Ready" ("t") _RT_Instrument_State."Shutting Down" ("t")] -> w951
                  tunnel: [u8 1 ("StartupMode") u8 2 ("StartupMode")] -> w950
                  frame False {
                    w954 = T22 2 items=["Same", "Empty", "VacFail", "Cancel", "CheckGas", "EleFail", "Probe1Fail", "Probe2Fail", "HeaterFail", "DoorOpen", "CheckComm", "PressStart", "StartRP"] ("Line2Msg (same)")
                    w955 = T23 5 items=["Same", "Empty", "Connected", "Starting", "Stopping", "Action", "On", "Service", "Call", "Acquiring", "Source"] ("Line1Msg (same)")
                    n518 = call "_RT Event.vi"("Event"="Going to Turbopump Ready state.") -> ()  [unwired: 2 in, 5 out]
                    n519 = call "_FPGA Set LCD Msg.vi"("ErrNum"="003", "Line2Msg (same)"=w954, "Line1Msg (same)"=w955) -> ()  [unwired: 4 in, 3 out]
                  }
                  frame True {
                  }
                }
                n520 = global write "_RT Global.vi" "StartupMode"(w950) -> ()
              }
              frame True {
                # "High Vacuum Achieved"
                n521 = case shown="False" w961 {
                  tunnel: [_RT_Instrument_State."Source Standby" ("t") _RT_Instrument_State."Going to Ready" ("t")] -> w966
                  frame False {
                    n522 = call "_RT Event.vi"("Event"="Going to Source Standby state.") -> ()  [unwired: 2 in, 5 out]
                    n523 = global write "_RT Global.vi" "StartupMode"(u8 1 ("StartupMode")) -> ()
                  }
                  frame True {
                    # "Source OK"
                  }
                }
                n524 = xnode "Read/Write Control"("FPGA VI Reference In"=w960, "FilaB"=FALSE) -> ("FPGA VI Reference Out"=w963:refnum<k20>, "error out"=w964:errorcluster)  [unwired: 1 in]
                n525 = xnode "Read/Write Control"("FPGA VI Reference In"=w963, "error in"=w964, "FilaC"=TRUE) -> ()  [unwired: 2 out]
              }
            }
          }
        }
      }
      frame "Going to Ready" {
        w974 = T22 1 items=["Same", "Empty", "VacFail", "Cancel", "CheckGas", "EleFail", "Probe1Fail", "Probe2Fail", "HeaterFail", "DoorOpen", "CheckComm", "PressStart", "StartRP"] ("Line2Msg (same)")
        w975 = T23 6 items=["Same", "Empty", "Connected", "Starting", "Stopping", "Action", "On", "Service", "Call", "Acquiring", "Source"] ("Line1Msg (same)")
        n526 = call "_FPGA Set LEDs.vi"("LED Command"=_LED_States."Off BRP") -> ("error out"=w977:errorcluster)  [unwired: 3 in, 3 out]
        n527 = call "_FPGA Set LEDs.vi"("error in (no error)"=w977, "LED Command"=_LED_States."Solid P") -> ("error out"=w979:errorcluster)  [unwired: 2 in, 3 out]
        n528 = call "_FPGA Set LCD Msg.vi"("error in"=w979, "Line2Msg (same)"=w974, "Line1Msg (same)"=w975) -> ("error out"=w982:errorcluster)  [unwired: 4 in, 2 out]
        n529 = call "_RT Event.vi"("Event"="Analyzer is Ready") -> ()  [unwired: 2 in, 5 out]
        n530 = call "_FPGA Send LCD.vi"("error in (no error)"=w982, "Command"=_RT_LED_Num."ReadKey" ("LED#")) -> ("error out"=w971:errorcluster)  [unwired: 3 in, 3 out]
        n531 = call "_FPGA Set Parameters.vi"("error in"=w971, "Set Zero (on)"=FALSE) -> ()  [unwired: 7 in, 3 out]
        n532 = global write "_RT Global.vi" "StartupMode"(u8 0 ("StartupMode")) -> ()
        n533 = local write "Ready"(TRUE ("Status LED")) -> ()
        n534 = local write "Fault"(FALSE ("Status LED")) -> ()
      }
      frame "Ready", Default {
        n535 = local read "Connected?"() -> (w995:bool)
        n536 = call "_FPGA Read Key.vi"() -> ("error out"=w986:errorcluster, "Key Pressed"=w992:bool)  [unwired: 5 in, 2 out]
        n537 = local read "RunMode"() -> (w987:i32)
        n538 = call "_FPGA System Polling.vi"("error in (no error)"=w986, "Connected?"=w995, "CurInstrState"=w994) -> ("Running"=w988:bool, "Next InstrState"=w993:T2)  [unwired: 1 in, 3 out]
        n539 = case shown="3, 6, 7" w987 {
          tunnel: [_ TRUE] -> w991
          frame 0, Default {
          }
          frame 3, 6, 7 {
          }
        }
        n540 = local write "Running"(w988) -> ()
        n541 = And(x=w991, y=w988) -> (x .and. y?=w990:bool)
        n542 = case shown="True" w990 {
          tunnel: [w998 _RT_Instrument_State."Running" ("InstrState")] -> w996
          tunnel: w993 -> [w1006 _]
          tunnel: w992 -> [w1004 _]
          tunnel: w989 -> [w1001 w1014]
          tunnel: w988 -> [w1003 _]
          tunnel: w987 -> [w1002 _]
          frame False {
            n543 = Select(t=_RT_Instrument_State."Shutting Down", s=w1004, f=w1006) -> (s? t:f=w998:T2)
            n544 = Not Equal?(x=w998, y=_RT_Instrument_State."Ready" ("t")) -> (x != y?=w1000:bool)
            n545 = case shown="True" w1000 {
              tunnel: w998 -> [_ w1010]
              tunnel: w1003 -> [_ w1009]
              tunnel: w1002 -> [_ w1008]
              tunnel: w1001 -> [_ w1007]
              frame False {
              }
              frame True {
                n546 = Format Into String(format string="Instr State transitioned from Ready to %s; FPGA Running = %s; Run Mode = %d; Loop = %d." ("Event"), w1010, w1009, w1008, w1007) -> (resulting string=w1011:string)  [unwired: 2 in, 1 out]
                n547 = call "_RT Event.vi"("Event"=w1011) -> ()  [unwired: 2 in, 5 out]
              }
            }
          }
          frame True {
            w1016 = T22 1 items=["Same", "Empty", "VacFail", "Cancel", "CheckGas", "EleFail", "Probe1Fail", "Probe2Fail", "HeaterFail", "DoorOpen", "CheckComm", "PressStart", "StartRP"] ("Line2Msg (same)")
            w1017 = T23 9 items=["Same", "Empty", "Connected", "Starting", "Stopping", "Action", "On", "Service", "Call", "Acquiring", "Source"] ("Line1Msg (same)")
            n548 = call "_FPGA Set LEDs.vi"("LED Command"=_LED_States."Solid B") -> ("error out"=w1018:errorcluster)  [unwired: 3 in, 3 out]
            n549 = Format Into String(format string="A run has started; Loop = %d." ("Event"), w1014) -> (resulting string=w1013:string)  [unwired: 2 in, 1 out]
            n550 = call "_FPGA Set LCD Msg.vi"("error in"=w1018, "Line2Msg (same)"=w1016, "Line1Msg (same)"=w1017) -> ()  [unwired: 4 in, 3 out]
            n551 = call "_RT Event.vi"("Event"=w1013) -> ()  [unwired: 2 in, 5 out]
          }
        }
      }
      frame "Source Standby" {
        n552 = global read "_RT Global.vi" "StartupMode"() -> (w1023:u8)
        n553 = case shown="Default" w1023 {
          tunnel: [w1033 _RT_Instrument_State."Shutting Down" ("InstrState") _RT_Instrument_State."Starting Up" ("InstrState")] -> w1022
          tunnel: w1021 -> [w1030 _ _]
          frame Default {
            # "Allow system to shut down from this state"
            n554 = local read "Connected?"() -> (w1032:bool)
            n555 = call "_FPGA Read Key.vi"("CurStartupMode (0)"=u8 1) -> ("error out"=w1026:errorcluster, "Key Pressed"=w1035:bool)  [unwired: 4 in, 2 out]
            n556 = call "_FPGA System Polling.vi"("error in (no error)"=w1026, "Waiting (F)"=TRUE, "Connected?"=w1032, "CurInstrState"=w1030) -> ("Running"=w1031:bool, "Next InstrState"=w1029:T2)  [unwired: 1 in, 2 out]
            n557 = local write "Running"(w1031) -> ()
            n558 = Select(t=_RT_Instrument_State."Shutting Down", s=w1035, f=w1029) -> (s? t:f=w1033:T2)
          }
          frame 2 {
            # "Received a shutdown command"
          }
          frame 0 {
            # "Received a startup command"
          }
        }
        n559 = local write "Fault"(TRUE ("Status LED")) -> ()
        n560 = local write "Ready"(FALSE ("Status LED")) -> ()
      }
      frame "Running" {
        n561 = local read "Connected?"() -> (w1039:bool)
        n562 = call "_FPGA System Polling.vi"("Connected?"=w1039, "CurInstrState"=w1040) -> ("Running"=w1041:bool, "Next InstrState"=w1042:T2)  [unwired: 3 in, 2 out]
        n563 = local write "Running"(w1041) -> ()
        n564 = case shown="False" w1041 {
          tunnel: [_RT_Instrument_State."Ready" ("InstrState") w1057] -> w1043
          tunnel: w1042 -> [_ w1057]
          tunnel: w1040 -> [_ w1059]
          tunnel: w1038 -> [_ _]
          frame False {
            w1044 = T22 1 items=["Same", "Empty", "VacFail", "Cancel", "CheckGas", "EleFail", "Probe1Fail", "Probe2Fail", "HeaterFail", "DoorOpen", "CheckComm", "PressStart", "StartRP"] ("Line2Msg (same)")
            w1045 = T23 6 items=["Same", "Empty", "Connected", "Starting", "Stopping", "Action", "On", "Service", "Call", "Acquiring", "Source"] ("Line1Msg (same)")
            n565 = call "_FPGA Set LEDs.vi"("LED Command"=_LED_States."Off BRP") -> ("error out"=w1046:errorcluster)  [unwired: 3 in, 3 out]
            n566 = local write "Fault"(FALSE ("Status LED")) -> ()
            n567 = call "_FPGA Set LEDs.vi"("error in (no error)"=w1046, "LED Command"=_LED_States."Solid P") -> ("error out"=w1048:errorcluster)  [unwired: 2 in, 3 out]
            n568 = local write "Ready"(TRUE ("Status LED")) -> ()
            n569 = call "_FPGA Set LCD Msg.vi"("error in"=w1048, "Line2Msg (same)"=w1044, "Line1Msg (same)"=w1045) -> ("error out"=w1049:errorcluster)  [unwired: 4 in, 2 out]
            n570 = call "_RT Event.vi"("Event"="A run ended normally, analyzer is ready") -> ()  [unwired: 2 in, 5 out]
            n571 = call "_FPGA Send LCD.vi"("error in (no error)"=w1049, "Command"=_RT_LED_Num."ReadKey" ("LED#")) -> ()  [unwired: 3 in, 4 out]
            n572 = global write "_RT Global.vi" "StartupMode"(u8 0 ("StartupMode")) -> ()
          }
          frame True {
            n573 = Not Equal?(x=w1059, y=w1057) -> (x != y?=w1058:bool)
            n574 = case shown="True" w1058 {
              tunnel: w1057 -> [_ w1063]
              frame False {
              }
              frame True {
                w1064 = u16 0 ("Address")
                # "End a Run"
                n575 = Format Into String(format string="A run unexpectedly ended as RT state changed from Running to %s.", w1063) -> (resulting string=w1061:string)  [unwired: 2 in, 1 out]
                n576 = call "_FPGA Set LEDs.vi"("LED Command"=_LED_States."Off B") -> ("error out"=w1060:errorcluster)  [unwired: 3 in, 3 out]
                n577 = call "_RT Event.vi"("Event"=w1061) -> ()  [unwired: 2 in, 5 out]
                n578 = call "_FPGA Write Data.vi"("error in"=w1060, "Data"=w1064, "Address"=w1064) -> ()  [unwired: 3 in, 3 out]
              }
            }
          }
        }
      }
      frame "Lost Communication" {
        # "Allow system to shutdown from this state"
        n579 = local read "Connected?"() -> (w1074:bool)
        n580 = call "_FPGA Read Key.vi"("CurStartupMode (0)"=u8 1) -> ("error out"=w1066:errorcluster, "Key Pressed"=w1068:bool)  [unwired: 4 in, 2 out]
        n581 = call "_FPGA System Polling.vi"("error in (no error)"=w1066, "Connected?"=w1074, "CurInstrState"=w1073) -> ("Running"=w1072:bool, "Next InstrState"=w1071:T2)  [unwired: 2 in, 2 out]
        n582 = local write "Running"(w1072) -> ()
        n583 = Select(t=_RT_Instrument_State."Shutting Down", s=w1068, f=w1071) -> (s? t:f=w1070:T2)
      }
      frame "Shutting Down" {
        n584 = global read "_RT Global.vi" "StartupMode"() -> (w1080:u8)
        n585 = local read "Fault"() -> (w1088:bool)
        n586 = Greater Than 0?(x=w1080) -> (x > 0?=w1085:bool)
        n587 = Or(x=w1088, y=w1085) -> (x .or. y?=w1087:bool)
        n588 = Equal?(x=w1080, y=u8 1) -> (x = y?=w1078:bool)
        n589 = Select(t="Going to Roughing Pump Ready" ("Event"), s=w1078, f="Stopping Analyzer" ("Event")) -> (s? t:f=w1075:string)
        n590 = call "_RT Event.vi"("Event"=w1075) -> ("error out"=w1083:errorcluster)  [unwired: 2 in, 4 out]
        n591 = call "_Update Shutting Down.vi"("error in (no error)"=w1083, "Fault"=w1087) -> ("error Out"=w1081:errorcluster, "InstrState"=w1084:T2)  [unwired: 1 in, 3 out]
        n592 = call "_FPGA Send LCD.vi"("error in (no error)"=w1081, "Command"=_RT_LED_Num."ReadKey" ("LED#")) -> ()  [unwired: 2 in, 5 out]
        n593 = local write "Ready"(FALSE ("Status LED")) -> ()
      }
      frame "Fault" {
        # "Level 1 failure found and perform a total shutdown"
        n594 = stacked-sequence {
          frame #0 {
            n595 = local write "Ready"(FALSE ("Status LED")) -> ()
            n596 = call "_FPGA Set LEDs.vi"("LED Command"=_LED_States."Solid R") -> ()  [unwired: 3 in, 4 out]
            n597 = local write "Fault"(TRUE ("Status LED")) -> ()
            n598 = Wait (ms)(milliseconds to wait=u32 1800) -> ()  [unwired: 1 out]
          }
          frame #1 {
            n599 = call "_FPGA Send LCD.vi"("Command"=_RT_LED_Num."ReadKey" ("LED#")) -> ()  [unwired: 4 in, 4 out]
            n600 = global write "_RT Global.vi" "StartupMode"(u8 2 ("StartupMode")) -> ()
          }
        }
      }
    }
    n601 = global write "_RT Global.vi" "InstrState"(w791) -> ()
    n602 = Wait (ms)(milliseconds to wait=u32 280) -> ()  [unwired: 1 out]
    "InstrState" <- w791
  }
  n603 = Get Date/Time In Seconds() -> (seconds since 1Jan1904=w27:timestamp)
  n604 = To Double Precision Float(number=w27) -> (double precision float=w13:dbl)
  n605 = while {
    tunnel: w13 -> [w1096]
    stop <- FALSE stop-if-true
    # "Control the User1 indicator"
    n606 = Get Date/Time In Seconds() -> (seconds since 1Jan1904=w1097:timestamp)
    n607 = To Double Precision Float(number=w1097) -> (double precision float=w1098:dbl)
    n608 = Subtract(x=w1098, y=w1096) -> (x-y=w1099:dbl)
    "Time (s)" <- w1099
    n609 = global write "_RT Global.vi" "RT Time(s)"(w1099) -> ()
    n610 = local read "Connected?"() -> (w1104:bool)
    n611 = Select(t=u32 1800 ("milliseconds to wait"), s=w1104, f=u32 280 ("milliseconds to wait")) -> (s? t:f=w1106:u32)
    n612 = call <vilib>:"RT LEDs.vi"("State"=3, "LED Num"=0) -> ()  [unwired: 4 in, 2 out]
    n613 = Wait (ms)(milliseconds to wait=w1106) -> ()  [unwired: 1 out]
  }
